vi "Main5states_decoupled.vi"() -> ()   [LabVIEW 2021]
uses:
  controls/SynchroCheckCentral.ctl
  controls/SynchroCheckCentral_Info.ctl
  controls/SynchroCheckCentral_Data.ctl
  controls/3ph Phasor.ctl
  controls/Phasor.ctl
  controls/AFE_froming_Central.ctl
  controls/AFE_froming_Central_Info.ctl
  controls/AFE_froming_Central_Data.ctl
  controls/references.ctl
  controls/Connected_OPF.ctl
  controls/Connected_OPF_Info.ctl
  controls/Connected_OPF_Data.ctl
  controls/PVemulator_Central.ctl
  controls/PVemulator_Central_Info.ctl
  controls/PVemulator_Central_Data.ctl
  controls/measurements.ctl
  controls/measurements_SC.ctl
  controls/SC_references.ctl
  controls/MeteoBoxCentral.ctl
  controls/MeteoBoxCentral_Info.ctl
  controls/MeteoBoxCentral_Data.ctl
  controls/SCADA_to_SM.ctl
  controls/SCADAOGCentral_Info.ctl
  controls/SCADA_to_SM_Data.ctl
  controls/State Machine.ctl
  <vilib>/Platform/TimedLoop/XDataNode/timing_clust.ctl
  <vilib>/Platform/TimedLoop/XDataNode/nitl_modes.ctl
  <vilib>/Platform/TimedLoop/XDataNode/wakeup.ctl
  controls/PV_facade_central.ctl
  controls/PV_facade_cental_Info.ctl
  controls/PV_facade_central_Data.ctl
  controls/state_2.ctl
  <vilib>/Analysis/baseanly.llb/Mean (DBL).vi
  <vilib>/JDP Science/JSONtext/Next JSON Value.vi
  <vilib>/JDP Science/JSONtext/String Subset.vi
  <vilib>/JDP Science/JSONtext/Parsing/Advance past next JSON Value (inlined COPY).vi
  <vilib>/JDP Science/JSONtext/Parsing/Advance past whitespace.vi
  <vilib>/JDP Science/JSONtext/Parsing/Advance past String.vi
  <vilib>/JDP Science/JSONtext/Parsing/Advance past Number.vi
  <vilib>/JDP Science/JSONtext/Parsing/Advance past Line Ending.vi
  <vilib>/Utility/file.llb/Read Delimited Spreadsheet (DBL).vi
  <vilib>/JDP Science/JSONtext/Parsing/Parse Full Path or Item Name.vi
  <vilib>/JDP Science/JSONtext/Parsing/Advance past Array.vi
  <vilib>/JDP Science/JSONtext/Parsing/Advance past Object.vi
  <vilib>/JDP Science/JSONtext/support/Error Cluster From Code.vi
  <vilib>/JDP Science/JSONtext/Offset/Find Item Locations by Path.vi
  <vilib>/Platform/TimedLoop/XDataNode/XDataNode.xnode
  <vilib>/JDP Science/JSONtext/JSONtext.lvlib
  <userlib>/_OpenG.lib/boolean/boolean.llb/openg_boolean__ogtk.lvlib
  <vilib>/Platform/TimedLoop/XDataNode/XDNodeRunTimeDep.lvlib
  <vilib>/Analysis/NI_AALBase.lvlib
panel:
  out "old_sp_island_bool":bool=TRUE
  out "old_sp_island":dbl[](array[numeric])
  out "V_freq_for_island":dbl
  out "V_freq":dbl
  out "V angle":cluster{"output":dbl}(graph)
  in  "Reset_angle":bool
  out "SOC":cluster{"mean":dbl}(graph)
  out "V_control_fix_for_island":dbl
  out "V control":cluster{"output":dbl}(graph)
  out "V_control":dbl
  out "V_afe":dbl
  out "V_upstream":dbl
  in  "Reset_magnitude":bool
  out "SCADA data":bool
  in  "SCADA":T1={"Info"={"Resource"="MeteoBox", "Problem"=FALSE, "Timestamp"=0.0}, "Data"={"Voltage mag"=[], "Voltage angle"=[]}}
  in  "to connected-island":bool
  in  "Real_SOC":bool
  out "P_pv_facade":dbl
  in  "SOC":dbl=50.0
  in  "IN Meteo":T4={"Info"={"Resource"="MeteoBox", "Problem"=FALSE, "Timestamp"=0.0}, "Data"={"GI"=0.0, "GHI"=0.0, "GVI"=0.0, "Tair"=0.0, "Tcell roof"=0.0, "Global_Total_Irr"=0.0, "Diffused_Irr"=0.0, "Tcell facade"=0.0, "PV_mpp"={"perun"=0.0, "solarmax"=0.0, "facade"=0.0, "emul4"=0.0, "emul5"=0.0, "emul6"=0.0, "emul7"=0.0}}}
  out "SC_soc":dbl
  out "delta angle":dbl
  in  "Send sp DC?":bool
  in  "Send sp AC?":bool
  out "Zenone_Q":dbl
  out "Zenone_P":dbl
  out "forming SC?":bool
  out "OUT PV+SC":T7={"Info"={"Resource"="Zenone", "Problem"=FALSE, "Timestamp"=0.0}, "Data"={"Status 1"=FALSE, "Status 2"=FALSE, "measurements"={"V_PV1"=0.0, "V_CAP1"=0.0, "V_PV2"=0.0, "V_CAP2"=0.0, "V_grid2"=0.0, "V_PV3"=0.0, "V_CAP3"=0.0, "V_grid3"=0.0, "V_PV4"=0.0, "V_CAP4"=0.0, "V_grid4"=0.0, "V_grid1"=0.0, "P1"=0.0, "P2"=0.0, "P3"=0.0, "P4"=0.0}, "Status 3"=FALSE, "Status 4"=FALSE, "measurements SC"={"V_SC"=0.0, "V_CAP"=0.0, "V_grid"=0.0, "P"=0.0, "SOC"=0.0}, "Status SC"=FALSE, "Forming/Following"=FALSE, "Start forming"=FALSE, "SC references"={"Vdc"=0.0, "Pdc"=0.0}, "Start following"=FALSE}}
  out "PV data":bool
  out "AFE data":bool
  out "synchro data":bool
  in  "IN PV+SC":T7={"Info"={"Resource"="Zenone", "Problem"=FALSE, "Timestamp"=0.0}, "Data"={"Status 1"=FALSE, "Status 2"=FALSE, "measurements"={"V_PV1"=0.0, "V_CAP1"=0.0, "V_PV2"=0.0, "V_CAP2"=0.0, "V_grid2"=0.0, "V_PV3"=0.0, "V_CAP3"=0.0, "V_grid3"=0.0, "V_PV4"=0.0, "V_CAP4"=0.0, "V_grid4"=0.0, "V_grid1"=0.0, "P1"=0.0, "P2"=0.0, "P3"=0.0, "P4"=0.0}, "Status 3"=FALSE, "Status 4"=FALSE, "measurements SC"={"V_SC"=0.0, "V_CAP"=0.0, "V_grid"=0.0, "P"=0.0, "SOC"=0.0}, "Status SC"=FALSE, "Forming/Following"=FALSE, "Start forming"=FALSE, "SC references"={"Vdc"=0.0, "Pdc"=0.0}, "Start following"=FALSE}}
  out "iOPF data":bool
  out "cOPF data":bool
  in  "IN AFE":T13={"Info"={"Resource"="Zenone", "Problem"=FALSE, "Timestamp"=0.0}, "Data"={"Start forming 1"=FALSE, "Forming/Following"=[], "Start forming 2"=FALSE, "measurements"={"Vdc1"=0.0, "P1"=0.0, "Vdc2"=0.0, "P2"=0.0, "Q2"=0.0, "Vdc3"=0.0, "P3"=0.0, "Q3"=0.0, "Vdc4"=0.0, "P4"=0.0, "Q4"=0.0, "Q1"=0.0}, "Status"=[], "references"={"Vdc1"=0.0, "Vdc2"=0.0, "Qac2"=0.0, "Vdc3"=0.0, "Qac3"=0.0, "Vdc4"=0.0, "Qac4"=0.0, "Qac1"=0.0, "V_arg2"=0.0, "V_abs2"=0.0, "V_abs1"=0.0, "V_arg1"=0.0, "freq1"=0.0, "freq2"=0.0}, "Start following 1"=FALSE, "Start following 2"=FALSE}}
  in  "IN cOPF":T17={"Info"={"Resource"="Zenone", "Problem"=0.0, "Timestamp"=0.0}, "Data"={"Operation_mode"="Grid connected", "solution_feasible"=0.0, "Optimal_slack"="AFE 1", "setpoints"=[], "upper_layer_grid_info"={"Frequency"=0.0, "Angle"=0.0, "Magnitude"=0.0}, "SC_soc"=0.0, "PV"={"perun"=0.0, "solarmax"=0.0, "facade"=0.0, "emul4"=0.0, "emul5"=0.0, "emul6"=0.0, "emul7"=0.0}, "P_pv_facade"=0.0}}
  in  "IN iOPF":T17={"Info"={"Resource"="Zenone", "Problem"=0.0, "Timestamp"=0.0}, "Data"={"Operation_mode"="Grid connected", "solution_feasible"=0.0, "Optimal_slack"="AFE 1", "setpoints"=[], "upper_layer_grid_info"={"Frequency"=0.0, "Angle"=0.0, "Magnitude"=0.0}, "SC_soc"=0.0, "PV"={"perun"=0.0, "solarmax"=0.0, "facade"=0.0, "emul4"=0.0, "emul5"=0.0, "emul6"=0.0, "emul7"=0.0}, "P_pv_facade"=0.0}}
  in  "IN synchro":T20={"Info"={"Resource"="SyncroCheck", "Problem"=FALSE, "Timestamp"=0.0}, "Data"={"close/open relay"=TRUE, "Operation mode"="Grid connected", "V_Downstream"={"Phase A"={"Frequency"=0.0, "Magnitude"=0.0, "Angle [Deg]"=0.0}, "Phase B"={"Frequency"=0.0, "Magnitude"=0.0, "Angle [Deg]"=0.0}, "Phase C"={"Frequency"=0.0, "Magnitude"=0.0, "Angle [Deg]"=0.0}, "Phase N"={"Frequency"=0.0, "Magnitude"=0.0, "Angle [Deg]"=0.0}}, "V_UpStream"={"Phase A"={"Frequency"=0.0, "Magnitude"=0.0, "Angle [Deg]"=0.0}, "Phase B"={"Frequency"=0.0, "Magnitude"=0.0, "Angle [Deg]"=0.0}, "Phase C"={"Frequency"=0.0, "Magnitude"=0.0, "Angle [Deg]"=0.0}, "Phase N"={"Frequency"=0.0, "Magnitude"=0.0, "Angle [Deg]"=0.0}}, "Synchronised?"=TRUE}}
  out "OUT iOPF":T17={"Info"={"Resource"="Zenone", "Problem"=0.0, "Timestamp"=0.0}, "Data"={"Operation_mode"="Grid connected", "solution_feasible"=0.0, "Optimal_slack"="AFE 1", "setpoints"=[], "upper_layer_grid_info"={"Frequency"=0.0, "Angle"=0.0, "Magnitude"=0.0}, "SC_soc"=0.0, "PV"={"perun"=0.0, "solarmax"=0.0, "facade"=0.0, "emul4"=0.0, "emul5"=0.0, "emul6"=0.0, "emul7"=0.0}, "P_pv_facade"=0.0}}
  out "OUT cOPF":T17={"Info"={"Resource"="Zenone", "Problem"=0.0, "Timestamp"=0.0}, "Data"={"Operation_mode"="Grid connected", "solution_feasible"=0.0, "Optimal_slack"="AFE 1", "setpoints"=[], "upper_layer_grid_info"={"Frequency"=0.0, "Angle"=0.0, "Magnitude"=0.0}, "SC_soc"=0.0, "PV"={"perun"=0.0, "solarmax"=0.0, "facade"=0.0, "emul4"=0.0, "emul5"=0.0, "emul6"=0.0, "emul7"=0.0}, "P_pv_facade"=0.0}}
  out "OUT AFE":T13={"Info"={"Resource"="Zenone", "Problem"=FALSE, "Timestamp"=0.0}, "Data"={"Start forming 1"=FALSE, "Forming/Following"=[], "Start forming 2"=FALSE, "measurements"={"Vdc1"=0.0, "P1"=0.0, "Vdc2"=0.0, "P2"=0.0, "Q2"=0.0, "Vdc3"=0.0, "P3"=0.0, "Q3"=0.0, "Vdc4"=0.0, "P4"=0.0, "Q4"=0.0, "Q1"=0.0}, "Status"=[], "references"={"Vdc1"=0.0, "Vdc2"=0.0, "Qac2"=0.0, "Vdc3"=0.0, "Qac3"=0.0, "Vdc4"=0.0, "Qac4"=0.0, "Qac1"=0.0, "V_arg2"=0.0, "V_abs2"=0.0, "V_abs1"=0.0, "V_arg1"=0.0, "freq1"=0.0, "freq2"=0.0}, "Start following 1"=FALSE, "Start following 2"=FALSE}}
  out "OUT Synchro":T20={"Info"={"Resource"="SyncroCheck", "Problem"=FALSE, "Timestamp"=0.0}, "Data"={"close/open relay"=TRUE, "Operation mode"="Grid connected", "V_Downstream"={"Phase A"={"Frequency"=0.0, "Magnitude"=0.0, "Angle [Deg]"=0.0}, "Phase B"={"Frequency"=0.0, "Magnitude"=0.0, "Angle [Deg]"=0.0}, "Phase C"={"Frequency"=0.0, "Magnitude"=0.0, "Angle [Deg]"=0.0}, "Phase N"={"Frequency"=0.0, "Magnitude"=0.0, "Angle [Deg]"=0.0}}, "V_UpStream"={"Phase A"={"Frequency"=0.0, "Magnitude"=0.0, "Angle [Deg]"=0.0}, "Phase B"={"Frequency"=0.0, "Magnitude"=0.0, "Angle [Deg]"=0.0}, "Phase C"={"Frequency"=0.0, "Magnitude"=0.0, "Angle [Deg]"=0.0}, "Phase N"={"Frequency"=0.0, "Magnitude"=0.0, "Angle [Deg]"=0.0}}, "Synchronised?"=TRUE}}
  out "setpoints":dbl[](array[numeric])
  in  "nb instances":i16=7
  out "optimal_slack":string(combo)="AFE 1"
  out "iOPF valid":bool
  out "forming AFE?":bool
  out "cOPF valid?":bool
  out "synchronised?":bool
  in  "to grid connection":bool
  in  "to prepare for grid connection":bool
  in  "to island":bool
  in  "Stop":bool
  in  "to prepare for island":bool
  # "32.58"
  # "Islanding Manoeuvre - State Machine"
  # "synchronised"
  # "opf connected OK"
  # "opf island OK"
  # "forming AFE?"
  # "forming SC?"
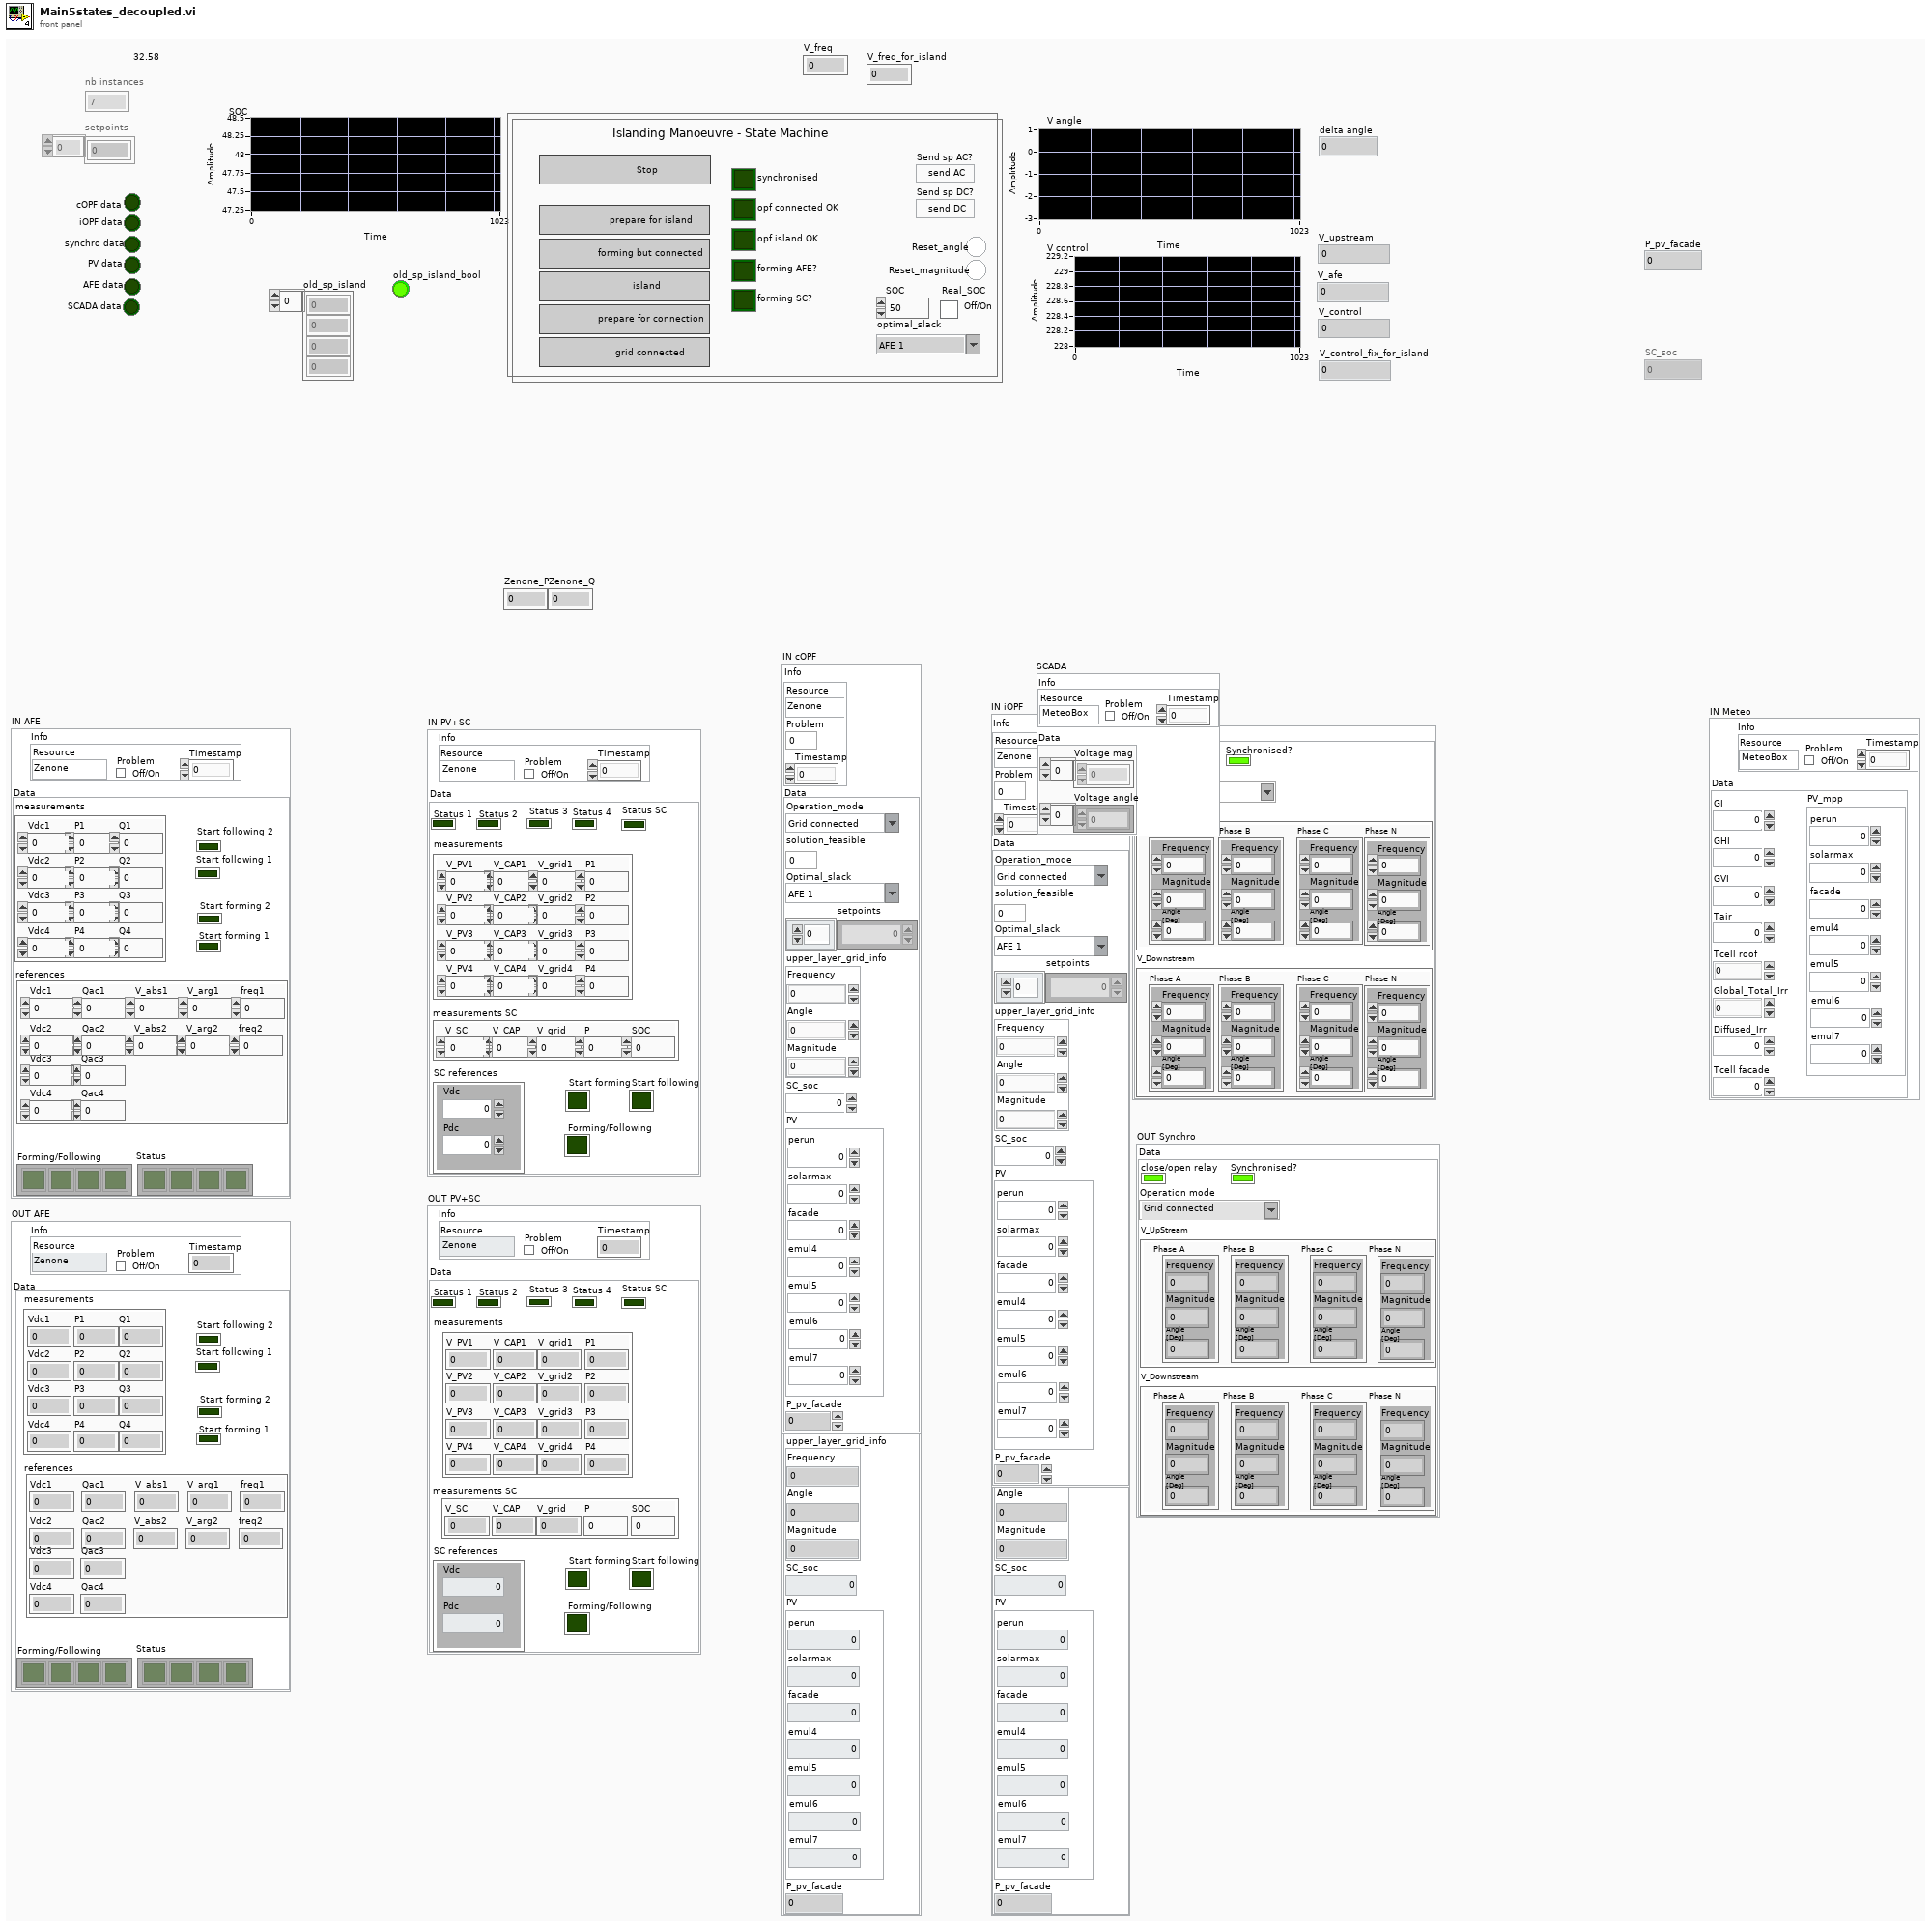
[diagram p1: front panel]
types:
  T1 = typedef "SCADA_to_SM.ctl" = cluster{"Info":T2, "Data":T3}
  T2 = typedef "SCADAOGCentral_Info.ctl" = cluster{"Resource":string, "Problem":bool, "Timestamp":dbl}
  T3 = typedef "SCADA_to_SM_Data.ctl" = cluster{"Voltage mag":dbl[], "Voltage angle":dbl[]}
  T4 = typedef "MeteoBoxCentral.ctl" = cluster{"Info":T5, "Data":T6}
  T5 = typedef "MeteoBoxCentral_Info.ctl" = cluster{"Resource":string, "Problem":bool, "Timestamp":dbl}
  T6 = typedef "MeteoBoxCentral_Data.ctl" = cluster{"GI":dbl, "GHI":dbl, "GVI":dbl, "Tair":dbl, "Tcell roof":dbl, "Global_Total_Irr":dbl, "Diffused_Irr":dbl, "Tcell facade":dbl, "PV_mpp":cluster{"perun":dbl, "solarmax":dbl, "facade":dbl, "emul4":dbl, "emul5":dbl, "emul6":dbl, "emul7":dbl}}
  T7 = typedef "PVemulator_Central.ctl" = cluster{"Info":T8, "Data":T9}
  T8 = typedef "PVemulator_Central_Info.ctl" = cluster{"Resource":string, "Problem":bool, "Timestamp":dbl}
  T9 = typedef "PVemulator_Central_Data.ctl" = cluster{"Status 1":bool, "Status 2":bool, "measurements":T10, "Status 3":bool, "Status 4":bool, "measurements SC":T11, "Status SC":bool, "Forming/Following":bool, "Start forming":bool, "SC references":T12, "Start following":bool}
  T10 = typedef "measurements.ctl" = cluster{"V_PV1":dbl, "V_CAP1":dbl, "V_PV2":dbl, "V_CAP2":dbl, "V_grid2":dbl, "V_PV3":dbl, "V_CAP3":dbl, "V_grid3":dbl, "V_PV4":dbl, "V_CAP4":dbl, "V_grid4":dbl, "V_grid1":dbl, "P1":dbl, "P2":dbl, "P3":dbl, "P4":dbl}
  T11 = typedef "measurements_SC.ctl" = cluster{"V_SC":dbl, "V_CAP":dbl, "V_grid":dbl, "P":dbl, "SOC":dbl}
  T12 = typedef "SC_references.ctl" = cluster{"Vdc":dbl, "Pdc":dbl}
  T13 = typedef "AFE_froming_Central.ctl" = cluster{"Info":T14, "Data":T15}
  T14 = typedef "AFE_froming_Central_Info.ctl" = cluster{"Resource":string, "Problem":bool, "Timestamp":dbl}
  T15 = typedef "AFE_froming_Central_Data.ctl" = cluster{"Start forming 1":bool, "Forming/Following":bool[], "Start forming 2":bool, "measurements":cluster{"Vdc1":dbl, "P1":dbl, "Vdc2":dbl, "P2":dbl, "Q2":dbl, "Vdc3":dbl, "P3":dbl, "Q3":dbl, "Vdc4":dbl, "P4":dbl, "Q4":dbl, "Q1":dbl}, "Status":bool[], "references":T16, "Start following 1":bool, "Start following 2":bool}
  T16 = typedef "references.ctl" = cluster{"Vdc1":dbl, "Vdc2":dbl, "Qac2":dbl, "Vdc3":dbl, "Qac3":dbl, "Vdc4":dbl, "Qac4":dbl, "Qac1":dbl, "V_arg2":dbl, "V_abs2":dbl, "V_abs1":dbl, "V_arg1":dbl, "freq1":dbl, "freq2":dbl}
  T17 = typedef "Connected_OPF.ctl" = cluster{"Info":T18, "Data":T19}
  T18 = typedef "Connected_OPF_Info.ctl" = cluster{"Resource":string, "Problem":dbl, "Timestamp":dbl}
  T19 = typedef "Connected_OPF_Data.ctl" = cluster{"Operation_mode":string, "solution_feasible":dbl, "Optimal_slack":string, "setpoints":dbl[], "upper_layer_grid_info":cluster{"Frequency":dbl, "Angle":dbl, "Magnitude":dbl}, "SC_soc":dbl, "PV":cluster{"perun":dbl, "solarmax":dbl, "facade":dbl, "emul4":dbl, "emul5":dbl, "emul6":dbl, "emul7":dbl}, "P_pv_facade":dbl}
  T20 = typedef "SynchroCheckCentral.ctl" = cluster{"Info":T21, "Data":T22}
  T21 = typedef "SynchroCheckCentral_Info.ctl" = cluster{"Resource":string, "Problem":bool, "Timestamp":dbl}
  T22 = typedef "SynchroCheckCentral_Data.ctl" = cluster{"close/open relay":bool, "Operation mode":string, "V_Downstream":T23, "V_UpStream":T23, "Synchronised?":bool}
  T23 = typedef "3ph Phasor.ctl" = cluster{"Phase A":T24, "Phase B":T24, "Phase C":T24, "Phase N":T24}
  T24 = typedef "Phasor.ctl" = cluster{"Frequency":dbl, "Magnitude":dbl, "Angle [Deg]":dbl}
  T25 = typedef "State Machine.ctl" = enum16{"Grid connected", "Prepare for island", "Forming but connected", "Island", "Prepare for connection"}
  T26 = typedef "XDNodeRunTimeDep.lvlib/timing_clust.ctl" = cluster{"Expected End [f-1]":u64, "Actual End [f-1]":u64, "Finished Late? [f-1]":bool, "Expected End [i-1]":u64, "Actual End [i-1]":u64, "Finished Late? [i-1]":bool, "Expected Start [i]":u64, "Actual Start [i]":u64, "Expected Start [f]":u64, "Actual Start [f]":u64, "Source Name":string, "Structure Name":string, "Period":i64, "Deadline":i64, "Offset":i64, "Start":i64, "Priority":i32, "Timeout":i32, "Mode":T27, "Wakeup Reason":T28, "Error":errorcluster, "Source Type":string, "Secondary Source Type":string, "Global End Time":u64, "Global Start Time":u64, "Frame Duration":u64, "Iteration Duration":u64, "Assigned CPU":i32, "I/O Scan Engine Mode":u32}
  T27 = typedef "XDNodeRunTimeDep.lvlib/nitl_modes.ctl" = enum32{"No Change", "Process missed periods, maintain original phase", "Discard missed periods, maintain original phase", "Process missed periods, ignore original phase", "Discard missed periods, ignore original phase"}
  T28 = typedef "XDNodeRunTimeDep.lvlib/wakeup.ctl" = enum32{"Normal", "Aborted", "Asynchronous wakeup", "Timing source error", "Timed loop error", "Timeout"}
  T29 = typedef "state_2.ctl" = string
  T30 = cluster{"Frequency":dbl, "Angle":dbl, "Magnitude":dbl}
  T31 = cluster{"perun":dbl, "solarmax":dbl, "facade":dbl, "emul4":dbl, "emul5":dbl, "emul6":dbl, "emul7":dbl}
  T32 = typedef "PV_facade_central.ctl" = cluster{"Info":T33, "Data":T34}
  T33 = typedef "PV_facade_cental_Info.ctl" = cluster{"Resource":string, "Problem":bool, "Timestamp":dbl}
  T34 = typedef "PV_facade_central_Data.ctl" = cluster{"P":dbl, "Q":dbl, "Pset":dbl, "Qset":dbl}
  T35 = typedef "Setpoints_CDA.ctl" = cluster{"ZENONE":T36, "BESS":T36, "PERUN":T36, "SOLMAX":T36}
  T36 = typedef "Setpoints_CDA_ZENONE.ctl" = cluster{"P_set [kW]":dbl, "Q_set [kVAr]":dbl}
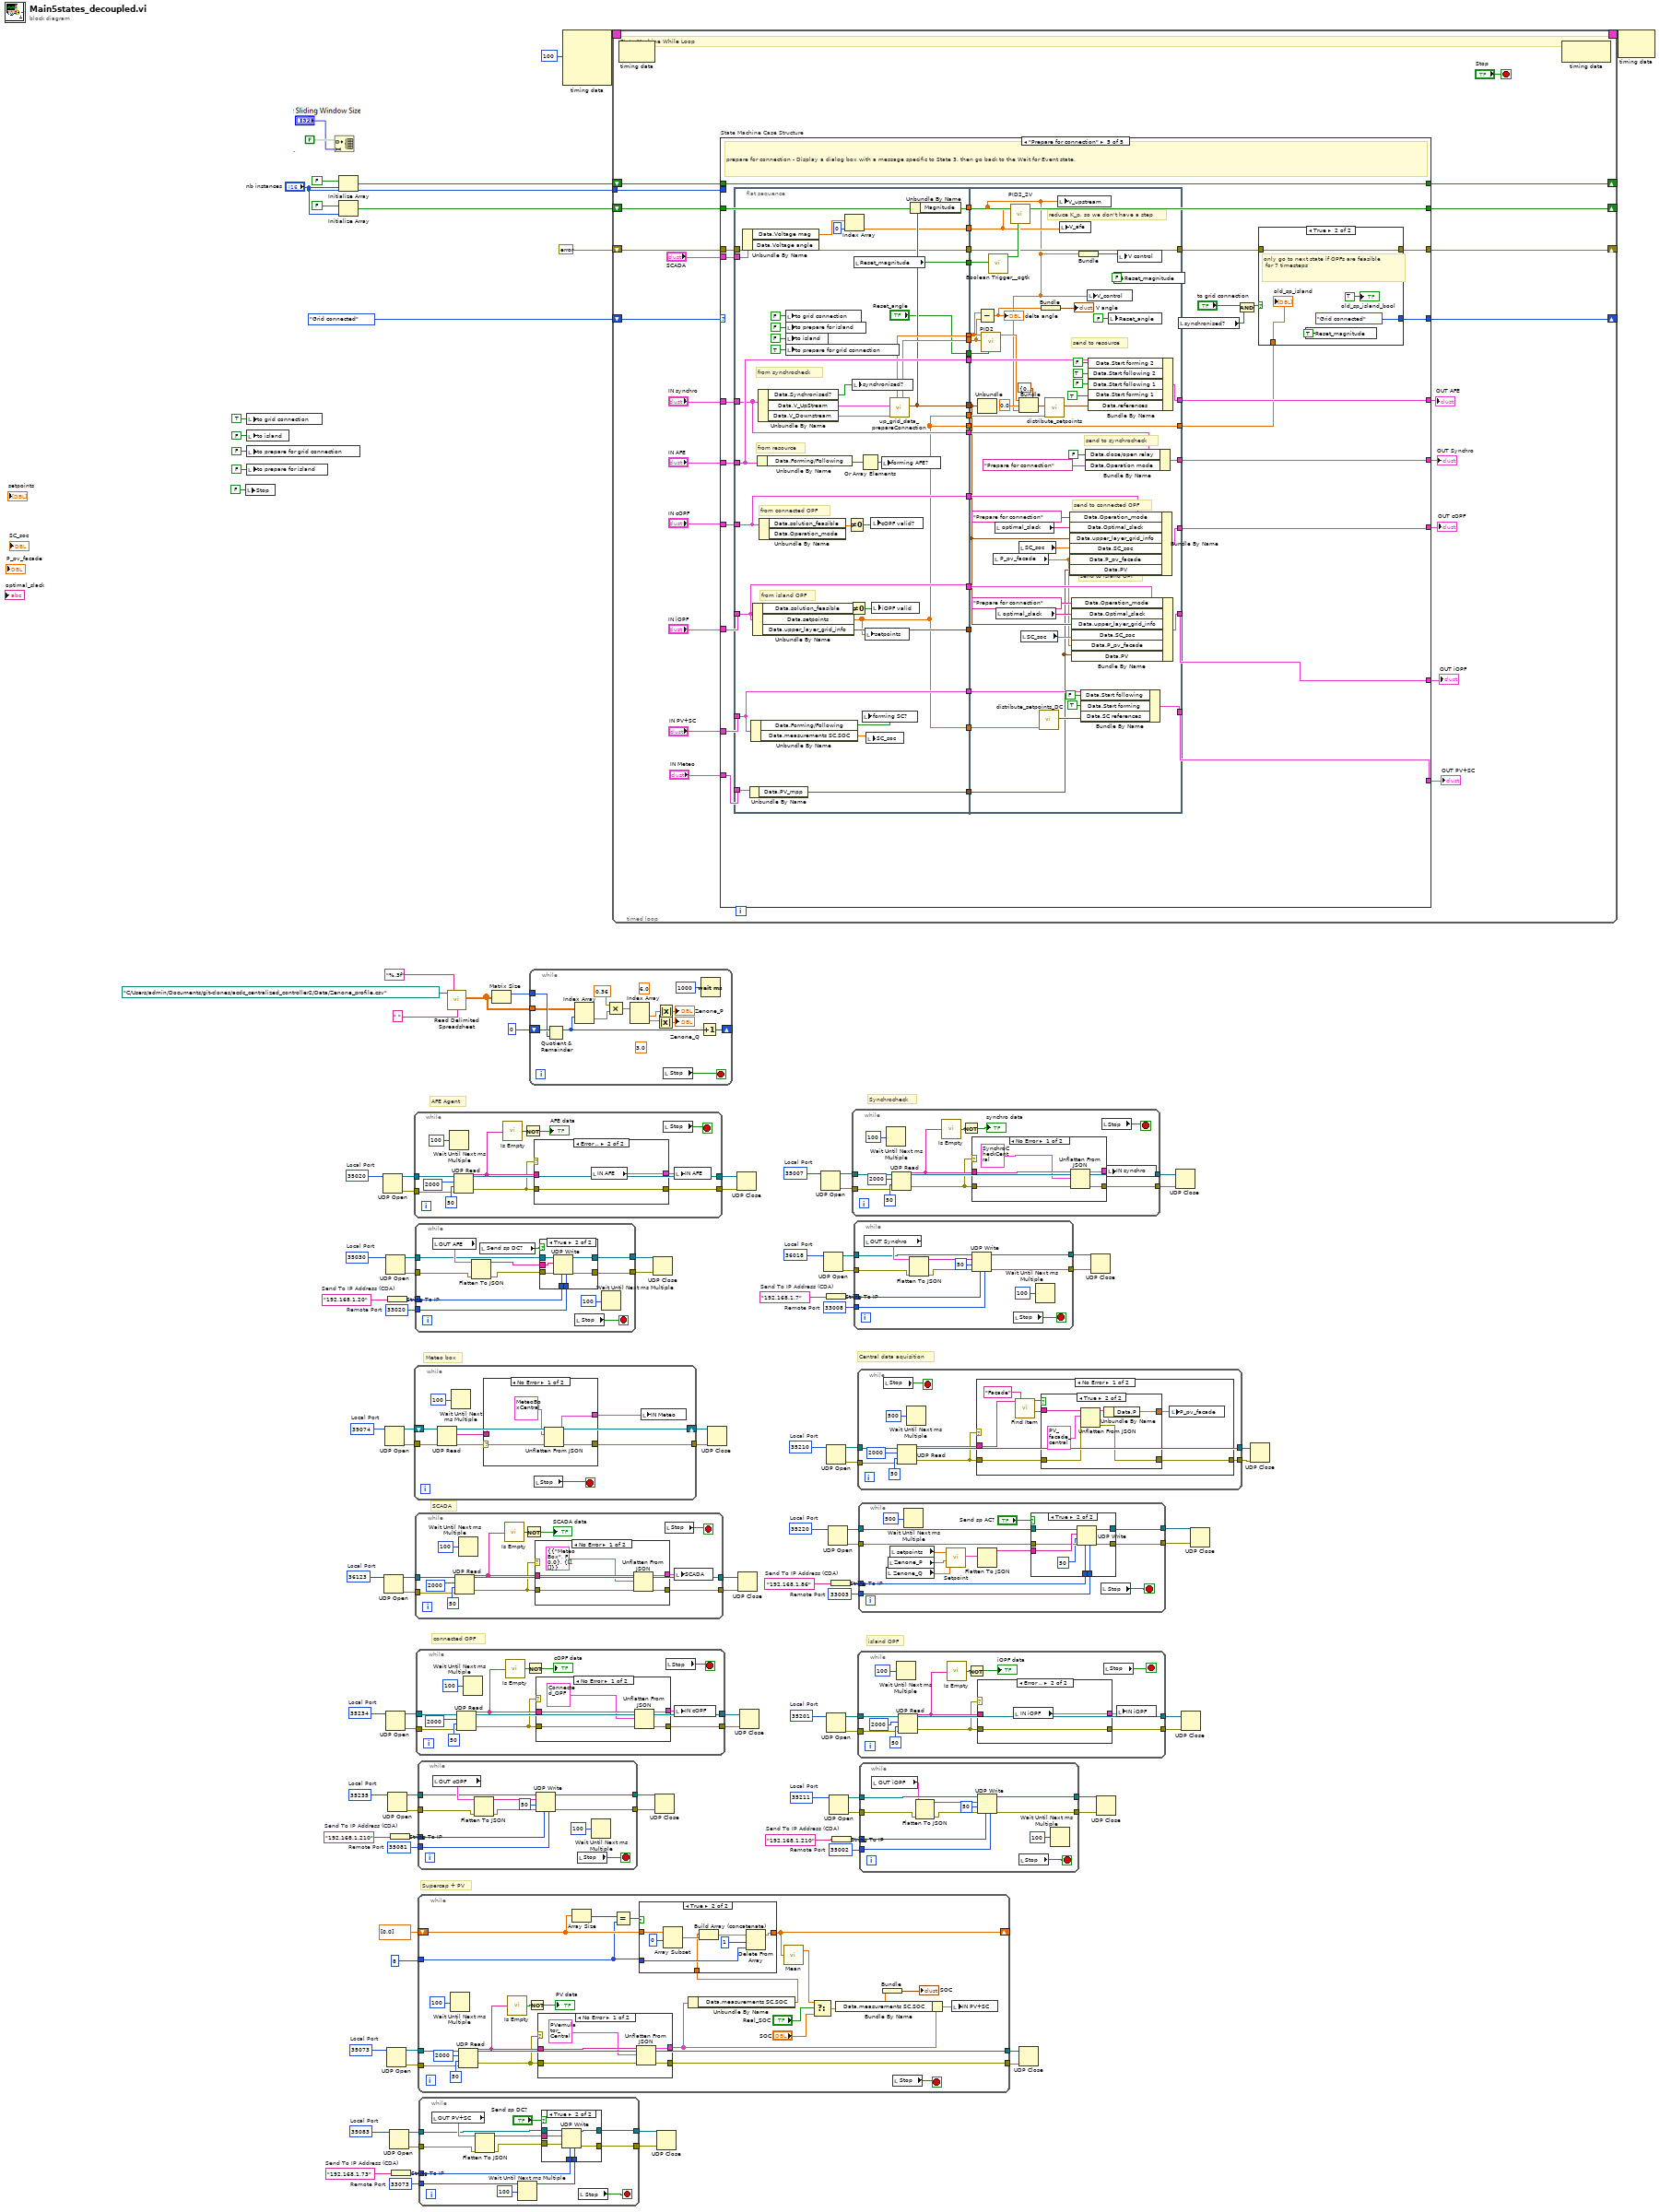
[diagram p0: block diagram]
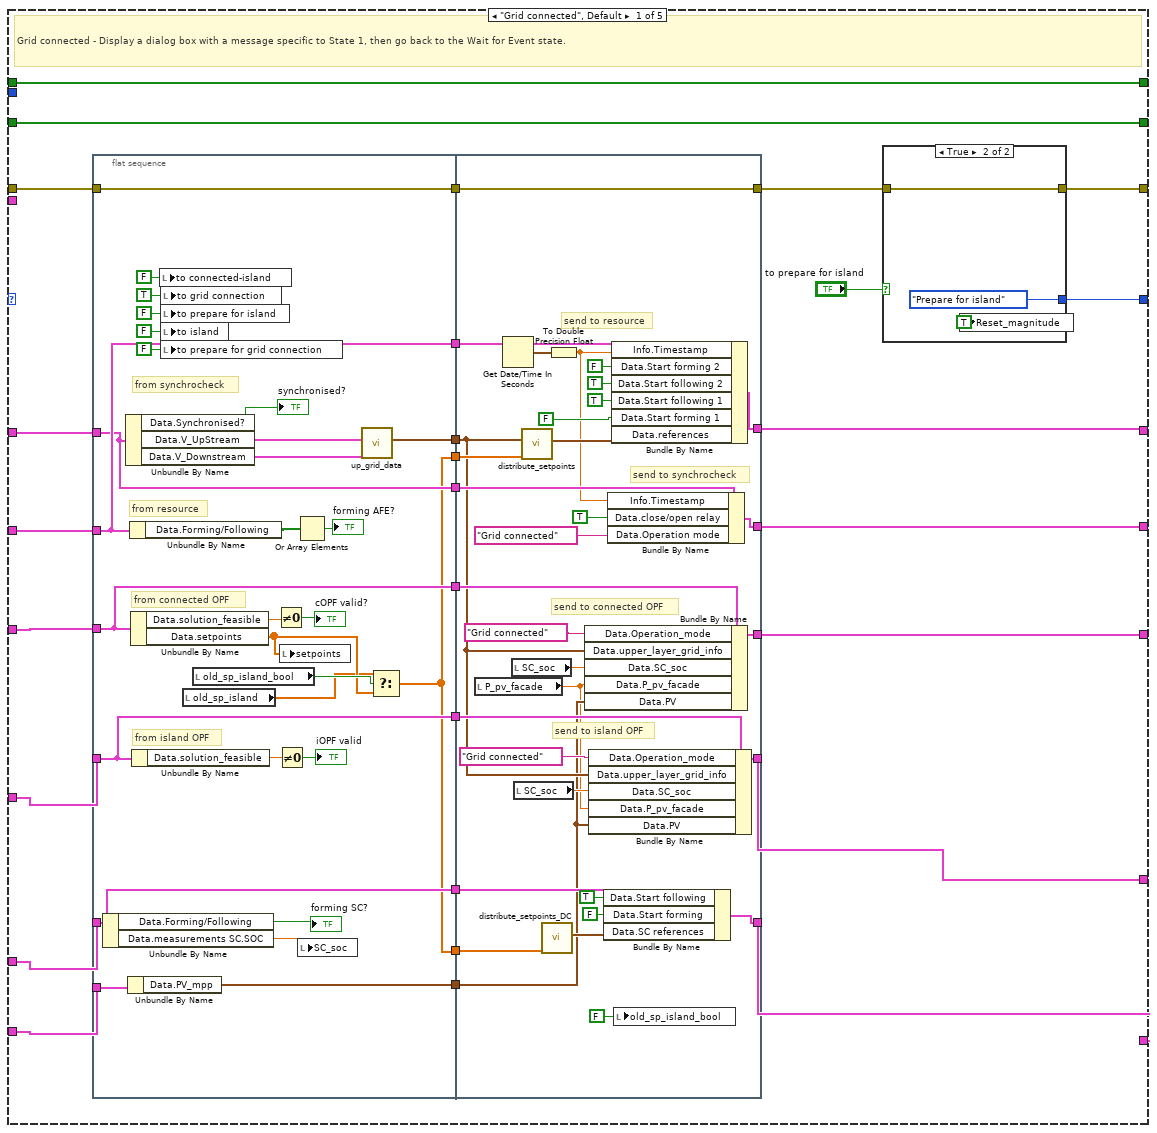
[diagram p2: hidden frame]
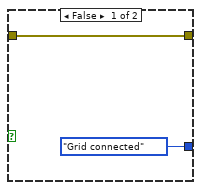
[diagram p3: hidden frame]
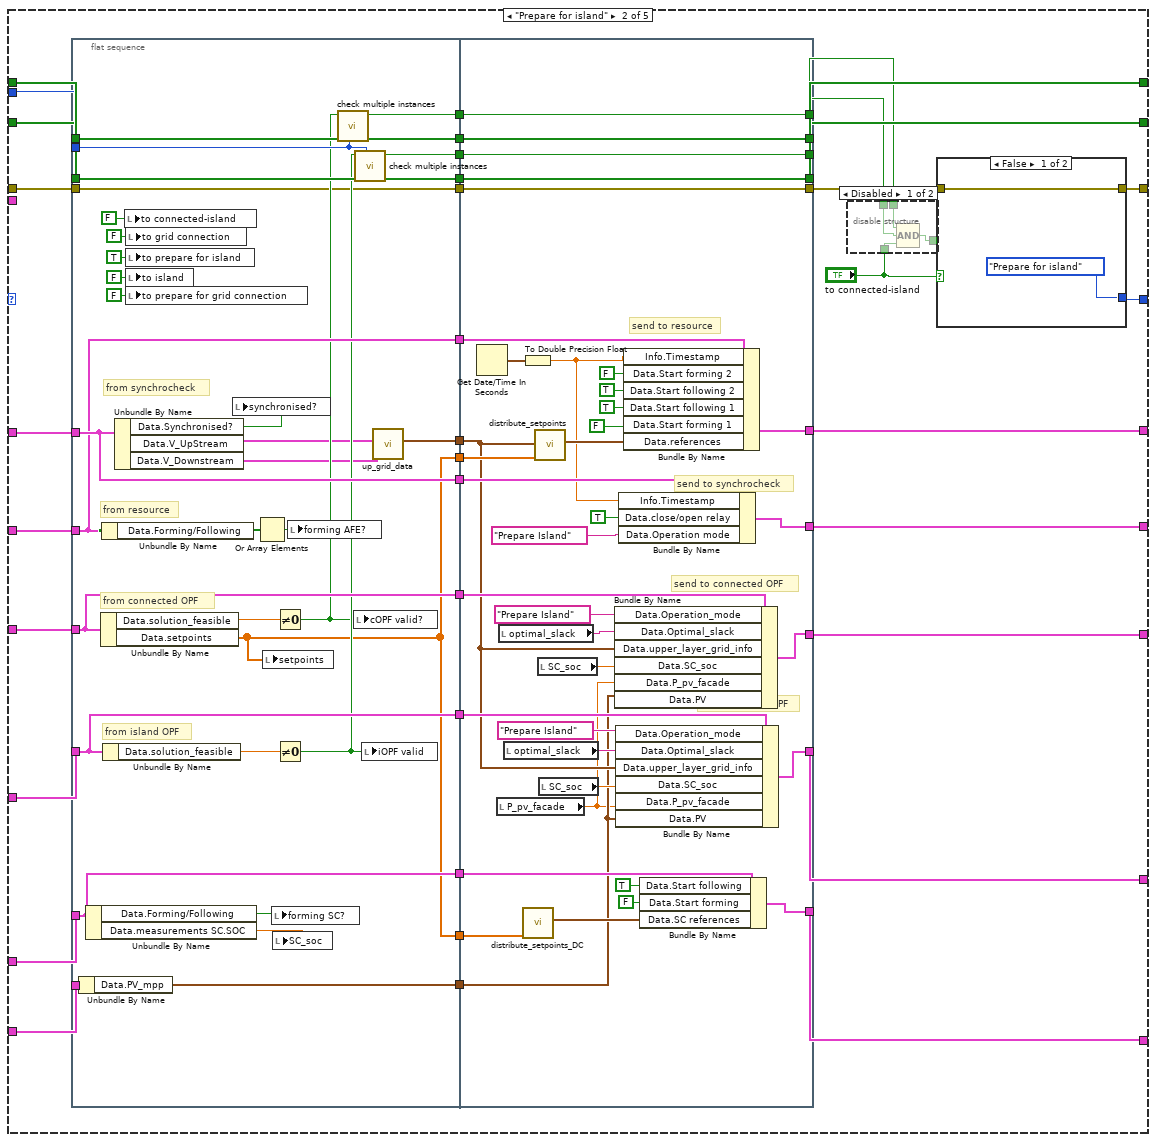
[diagram p4: hidden frame]
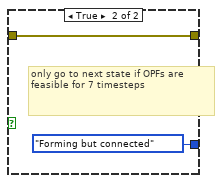
[diagram p6: hidden frame]
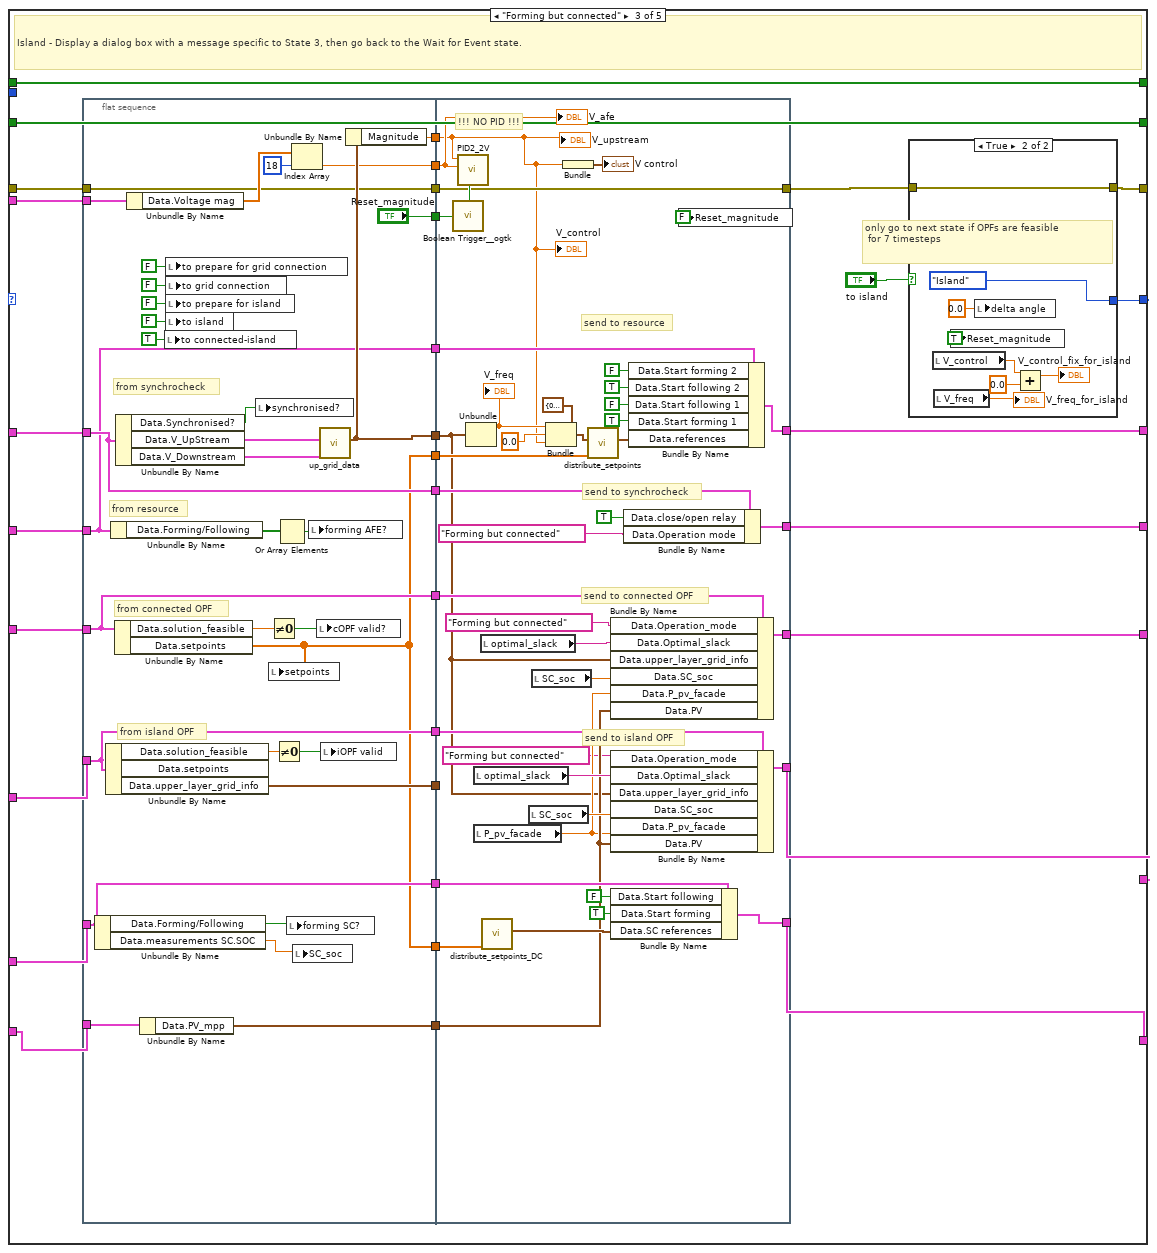
[diagram p7: hidden frame]
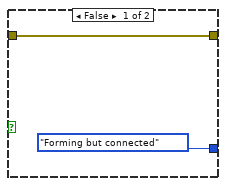
[diagram p8: hidden frame]
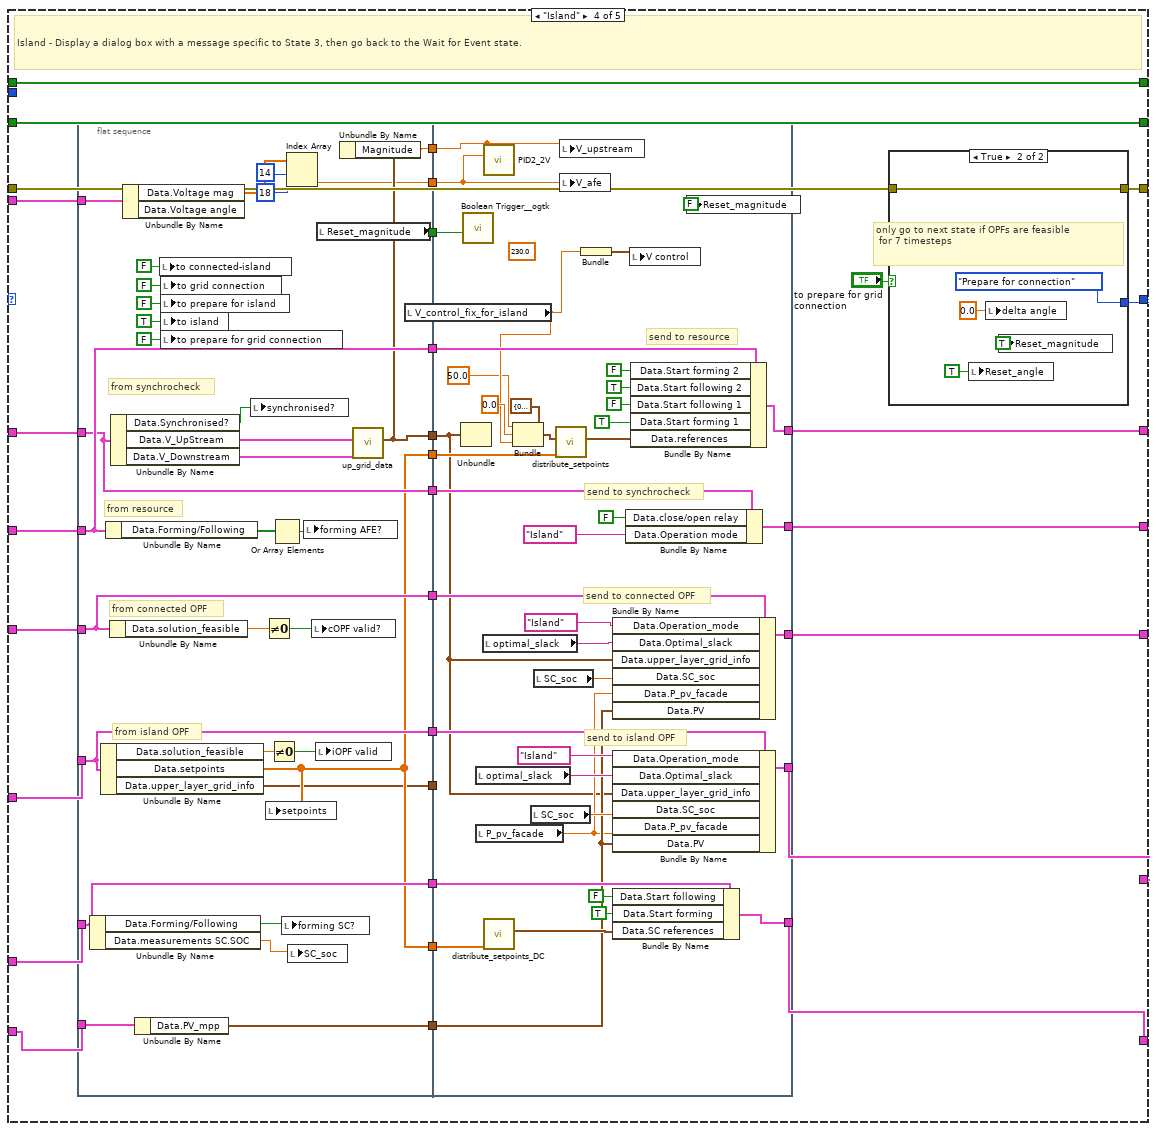
[diagram p9: hidden frame]
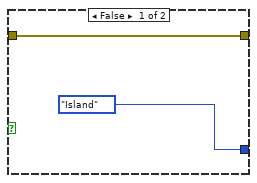
[diagram p10: hidden frame]
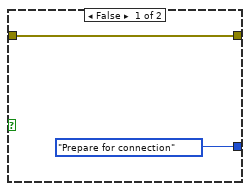
[diagram p11: hidden frame]
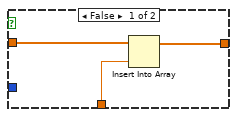
[diagram p12: hidden frame]
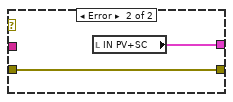
[diagram p13: hidden frame]
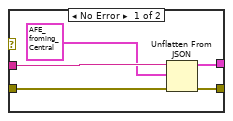
[diagram p16: hidden frame]
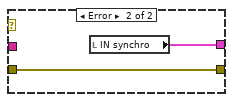
[diagram p17: hidden frame]
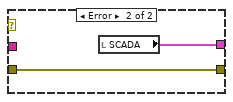
[diagram p18: hidden frame]
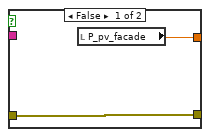
[diagram p20: hidden frame]
diagram:
  w10 = u16 35083  # Local Port
  w12 = u16 33073  # Remote Port
  w13 = "192.168.1.73"  # Send To IP Address (CDA)
  w14 = u16 35073  # Local Port
  w23 = u16 35030  # Local Port
  w25 = u16 33020  # Remote Port
  w26 = "192.168.1.20"  # Send To IP Address (CDA)
  w27 = u16 35020  # Local Port
  w35 = u16 36018  # Local Port
  w32 = u16 33008  # Remote Port
  w34 = "192.168.1.7"  # Send To IP Address (CDA)
  w33 = u16 35007  # Local Port
  w45 = u16 36123  # Local Port
  w54 = u16 35220  # Local Port
  w56 = u16 33003  # Remote Port
  w57 = "192.168.1.86"  # Send To IP Address (CDA)
  w58 = u16 35210  # Local Port
  w65 = u16 35211  # Local Port
  w63 = u16 35002  # Remote Port
  w64 = "192.168.1.210"  # Send To IP Address (CDA)
  w66 = u16 35201  # Local Port
  w80 = u16 35235  # Local Port
  w82 = u16 35081  # Remote Port
  w83 = "192.168.1.210"  # Send To IP Address (CDA)
  w84 = u16 35234  # Local Port
  w95 = u16 39074  # Local Port
  # "Supercap + PV"
  # "AFE Agent"
  # "Synchrocheck"
  # "SCADA"
  # "Meteo box"
  # "Central data aquisition"
  # "connected OPF"
  # "island OPF"
  n1 = local write "Stop"(FALSE ("Stop")) -> ()
  n2 = local write "to grid connection"(TRUE ("to grid connection")) -> ()
  n3 = local write "to island"(FALSE ("to island")) -> ()
  n4 = local write "to prepare for grid connection"(FALSE ("to prepare for grid connection")) -> ()
  n5 = local write "to prepare for island"(FALSE ("to prepare for island")) -> ()
  n6 = Initialize Array(FALSE, "nb instances") -> (w110:bool[])
  n7 = Initialize Array(FALSE, "nb instances") -> (w108:bool[])
  n8 = UDP Open(11:w27) -> (port=w29:refnum<k16>, 0:w28:errorcluster)  [unwired: 4 in, 1 out]
  n9 = UDP Open(11:w45) -> (port=w47:refnum<k16>, 0:w46:errorcluster)  [unwired: 4 in, 1 out]
  n10 = UDP Open(11:w95) -> (port=w94:refnum<k16>, 0:w93:errorcluster)  [unwired: 4 in, 1 out]
  n11 = UDP Open(11:w23) -> (port=w20:refnum<k16>, 0:w19:errorcluster)  [unwired: 4 in, 1 out]
  n12 = UDP Open(11:w84) -> (port=w86:refnum<k16>, 0:w85:errorcluster)  [unwired: 4 in, 1 out]
  n13 = UDP Open(11:w14) -> (port=w16:refnum<k16>, 0:w15:errorcluster)  [unwired: 4 in, 1 out]
  n14 = String To IP(1:w26) -> (0:w24:u32)
  n15 = UDP Open(11:w80) -> (port=w77:refnum<k16>, 0:w76:errorcluster)  [unwired: 4 in, 1 out]
  n16 = UDP Open(11:w10) -> (port=w7:refnum<k16>, 0:w6:errorcluster)  [unwired: 4 in, 1 out]
  n17 = String To IP(1:w83) -> (0:w81:u32)
  n18 = String To IP(1:w13) -> (0:w11:u32)
  n19 = while {
    tunnel: w29 -> [w119]
    tunnel: w28 -> [w118]
    tunnel: [w117] -> w31
    tunnel: [w116] -> w30
    stop <- w122 stop-if-true
    (unwired) i64 0 ("Iteration Duration")
    n20 = Wait Until Next ms Multiple(millisecond multiple=u32 100) -> ()  [unwired: 1 out]
    n21 = UDP Read(connection ID=w119, max size (548)=2000, timeout ms (25000)=50, 8:w118) -> (data out=w120:string, error out=w115:errorcluster, 3:w116:refnum<k16>)  [unwired: 2 out]
    n22 = call <vilib>:"Is Empty.vi"("JSON"=w120) -> ("Empty"=w123:bool)  [unwired: 4 in]
    n23 = Not(x=w123) -> (.not. x?=→"AFE data":bool)
    n24 = case shown="Error .." w115 {
      tunnel: w115 -> [w128 w131]
      tunnel: w120 -> [w127 _]
      tunnel: [w129 w131] -> w117
      tunnel: [w126 w130] -> w121
      frame No Error {
        n25 = Unflatten From JSON(JSON string=w127, type and defaults=T13 {"Info"={"Resource"="Zenone", "Problem"=FALSE, "Timestamp"=0.0}, "Data"={"Start forming 1"=FALSE, "Forming/Following"=[], "Start forming 2"=FALSE, "measurements"={"Vdc1"=0.0, "P1"=0.0, "Vdc2"=0.0, "P2"=0.0, "Q2"=0.0, "Vdc3"=0.0, "P3"=0.0, "Q3"=0.0, "Vdc4"=0.0, "P4"=0.0, "Q4"=0.0, "Q1"=0.0}, "Status"=[], "references"={"Vdc1"=0.0, "Vdc2"=0.0, "Qac2"=0.0, "Vdc3"=0.0, "Qac3"=0.0, "Vdc4"=0.0, "Qac4"=0.0, "Qac1"=0.0, "V_arg2"=0.0, "V_abs2"=0.0, "V_abs1"=0.0, "V_arg1"=0.0, "freq1"=0.0, "freq2"=0.0}, "Start following 1"=FALSE, "Start following 2"=FALSE}} ("IN AFE"), error in (no error)=w128) -> (value=w126:T13, error out=w129:errorcluster)  [unwired: 4 in]
      }
      frame Error {
        n26 = local read "IN AFE"() -> (w130:T13)
      }
    }
    n27 = local read "Stop"() -> (w122:bool)
    n28 = local write "IN AFE"(w121) -> ()
  }
  n29 = while {
    tunnel: w93 -> [w139]
    tunnel: [w136] -> w92
    shift-right: [w135] -> w91
    shift-left: w94 -> [w140]
    stop <- w134 stop-if-true
    n30 = UDP Read(connection ID=w140, 8:w139) -> (data out=w138:string, error out=w133:errorcluster, 3:w135:refnum<k16>)  [unwired: 2 in, 2 out]
    n31 = Wait Until Next ms Multiple(millisecond multiple=u32 100) -> ()  [unwired: 1 out]
    n32 = case shown="No Error" w133 {
      selector: w133 -> [w141 w146]
      tunnel: w138 -> [w145 _]
      tunnel: [w143 w147] -> w137
      tunnel: [w142 w146] -> w136
      frame No Error {
        n33 = Unflatten From JSON(JSON string=w145, type and defaults=T4 {"Info"={"Resource"="MeteoBox", "Problem"=FALSE, "Timestamp"=0.0}, "Data"={"GI"=0.0, "GHI"=0.0, "GVI"=0.0, "Tair"=0.0, "Tcell roof"=0.0, "Global_Total_Irr"=0.0, "Diffused_Irr"=0.0, "Tcell facade"=0.0, "PV_mpp"={"perun"=0.0, "solarmax"=0.0, "facade"=0.0, "emul4"=0.0, "emul5"=0.0, "emul6"=0.0, "emul7"=0.0}}} ("Cluster"), error in (no error)=w141) -> (value=w143:T4, error out=w142:errorcluster)  [unwired: 4 in]
      }
      frame Error {
        n34 = local read "IN Meteo"() -> (w147:T4)
      }
    }
    n35 = local read "Stop"() -> (w134:bool)
    n36 = local write "IN Meteo"(w137) -> ()
  }
  n37 = while {
    tunnel: w25 -> [w151]
    tunnel: w24 -> [w152]
    tunnel: w20 -> [w154]
    tunnel: w19 -> [w158]
    tunnel: [w150] -> w22
    tunnel: [w149] -> w21
    stop <- w157 stop-if-true
    n38 = local read "OUT AFE"() -> (w159:T13)
    n39 = Flatten To JSON(anything=w159, error in (no error)=w158) -> (JSON string=w155:string, 11:w153:errorcluster)  [unwired: 1 in]
    n40 = local read "Send sp DC?"() -> (w156:bool)
    n41 = case shown="True" w156 {
      tunnel: w155 -> [_ w168]
      tunnel: [w160 w167] -> w149
      tunnel: [w161 w166] -> w150
      tunnel: w154 -> [w161 w165]
      tunnel: w153 -> [w160 w162]
      tunnel: w152 -> [_ w164]
      tunnel: w151 -> [_ w163]
      frame False {
      }
      frame True {
        n42 = UDP Write(address=w164, port or service name=w163, connection ID=w165, data in=w168, 8:w162) -> (error out=w167:errorcluster, 3:w166:refnum<k16>)  [unwired: 1 in]
      }
    }
    n43 = local read "Stop"() -> (w157:bool)
    n44 = Wait Until Next ms Multiple(millisecond multiple=u32 100) -> ()  [unwired: 1 out]
  }
  n45 = while {
    tunnel: w47 -> [w177]
    tunnel: w46 -> [w176]
    tunnel: [w175] -> w49
    tunnel: [w174] -> w48
    stop <- w179 stop-if-true
    (unwired) i64 0 ("Iteration Duration")
    n46 = UDP Read(connection ID=w177, max size (548)=2000, timeout ms (25000)=50, 8:w176) -> (data out=w178:string, error out=w173:errorcluster, 3:w174:refnum<k16>)  [unwired: 2 out]
    n47 = Wait Until Next ms Multiple(millisecond multiple=u32 100) -> ()  [unwired: 1 out]
    n48 = call <vilib>:"Is Empty.vi"("JSON"=w178) -> ("Empty"=w180:bool)  [unwired: 4 in]
    n49 = Not(x=w180) -> (.not. x?=→"SCADA data":bool)
    n50 = case shown="No Error" w173 {
      tunnel: w173 -> [w185 w188]
      tunnel: w178 -> [w184 _]
      tunnel: [w186 w188] -> w175
      tunnel: [w183 w187] -> w171
      frame No Error {
        n51 = Unflatten From JSON(JSON string=w184, type and defaults=T1 {"Info"={"Resource"="MeteoBox", "Problem"=FALSE, "Timestamp"=0.0}, "Data"={"Voltage mag"=[], "Voltage angle"=[]}} ("Cluster"), error in (no error)=w185) -> (value=w183:T1, error out=w186:errorcluster)  [unwired: 4 in]
      }
      frame Error {
        n52 = local read "SCADA"() -> (w187:T1)
      }
    }
    n53 = local read "Stop"() -> (w179:bool)
    n54 = local write "SCADA"(w171) -> ()
  }
  n55 = while {
    tunnel: w86 -> [w195]
    tunnel: w85 -> [w194]
    tunnel: [w193] -> w88
    tunnel: [w192] -> w87
    stop <- w198 stop-if-true
    (unwired) i64 0 ("Iteration Duration")
    n56 = UDP Read(connection ID=w195, max size (548)=2000, timeout ms (25000)=50, 8:w194) -> (data out=w196:string, error out=w191:errorcluster, 3:w192:refnum<k16>)  [unwired: 2 out]
    n57 = Wait Until Next ms Multiple(millisecond multiple=u32 100) -> ()  [unwired: 1 out]
    n58 = call <vilib>:"Is Empty.vi"("JSON"=w196) -> ("Empty"=w200:bool)  [unwired: 4 in]
    n59 = Not(x=w200) -> (.not. x?=→"cOPF data":bool)
    n60 = case shown="No Error" w191 {
      tunnel: w191 -> [w205 w208]
      tunnel: w196 -> [w204 _]
      tunnel: [w206 w208] -> w193
      tunnel: [w202 w207] -> w197
      frame No Error {
        n61 = Unflatten From JSON(JSON string=w204, type and defaults=T17 {"Info"={"Resource"="Zenone", "Problem"=0.0, "Timestamp"=0.0}, "Data"={"Operation_mode"="Grid connected", "solution_feasible"=0.0, "Optimal_slack"="AFE 1", "setpoints"=[], "upper_layer_grid_info"={"Frequency"=0.0, "Angle"=0.0, "Magnitude"=0.0}, "SC_soc"=0.0, "PV"={"perun"=0.0, "solarmax"=0.0, "facade"=0.0, "emul4"=0.0, "emul5"=0.0, "emul6"=0.0, "emul7"=0.0}, "P_pv_facade"=0.0}} ("IN iOPF"), error in (no error)=w205) -> (value=w202:T17, error out=w206:errorcluster)  [unwired: 4 in]
      }
      frame Error {
        n62 = local read "IN cOPF"() -> (w207:T17)
      }
    }
    n63 = local read "Stop"() -> (w198:bool)
    n64 = local write "IN cOPF"(w197) -> ()
  }
  n65 = while {
    tunnel: w82 -> [w220]
    tunnel: w81 -> [w219]
    tunnel: w77 -> [w216]
    tunnel: w76 -> [w215]
    tunnel: [w214] -> w79
    tunnel: [w213] -> w78
    stop <- w212 stop-if-true
    n66 = local read "OUT cOPF"() -> (w217:T17)
    n67 = Flatten To JSON(anything=w217, error in (no error)=w215) -> (JSON string=w218:string, 11:w211:errorcluster)  [unwired: 1 in]
    n68 = UDP Write(address=w219, port or service name=w220, connection ID=w216, data in=w218, 8:w211, 9:50 ("timeout ms (25000)")) -> (error out=w213:errorcluster, 3:w214:refnum<k16>)
    n69 = local read "Stop"() -> (w212:bool)
    n70 = Wait Until Next ms Multiple(millisecond multiple=u32 100) -> ()  [unwired: 1 out]
  }
  n71 = while {
    tunnel: w16 -> [w241]
    tunnel: w15 -> [w240]
    tunnel: [w239] -> w18
    tunnel: [w238] -> w17
    tunnel: 8 ("millisecond multiple") -> [w225]
    shift-right: [w221] -> _
    shift-left: dbl[] [0.0] -> [w226]
    stop <- w243 stop-if-true
    (unwired) i64 0 ("Iteration Duration")
    n72 = Wait Until Next ms Multiple(millisecond multiple=u32 100) -> ()  [unwired: 1 out]
    n73 = UDP Read(connection ID=w241, max size (548)=2000, timeout ms (25000)=50, 8:w240) -> (data out=w242:string, error out=w237:errorcluster, 3:w238:refnum<k16>)  [unwired: 2 out]
    n74 = call <vilib>:"Is Empty.vi"("JSON"=w242) -> ("Empty"=w244:bool)  [unwired: 4 in]
    n75 = Not(x=w244) -> (.not. x?=→"PV data":bool)
    n76 = case shown="No Error" w237 {
      tunnel: w237 -> [w260 w263]
      tunnel: w242 -> [w259 _]
      tunnel: [w261 w263] -> w239
      tunnel: [w258 w262] -> w231
      frame No Error {
        n77 = Unflatten From JSON(JSON string=w259, type and defaults=T7 {"Info"={"Resource"="Zenone", "Problem"=FALSE, "Timestamp"=0.0}, "Data"={"Status 1"=FALSE, "Status 2"=FALSE, "measurements"={"V_PV1"=0.0, "V_CAP1"=0.0, "V_PV2"=0.0, "V_CAP2"=0.0, "V_grid2"=0.0, "V_PV3"=0.0, "V_CAP3"=0.0, "V_grid3"=0.0, "V_PV4"=0.0, "V_CAP4"=0.0, "V_grid4"=0.0, "V_grid1"=0.0, "P1"=0.0, "P2"=0.0, "P3"=0.0, "P4"=0.0}, "Status 3"=FALSE, "Status 4"=FALSE, "measurements SC"={"V_SC"=0.0, "V_CAP"=0.0, "V_grid"=0.0, "P"=0.0, "SOC"=0.0}, "Status SC"=FALSE, "Forming/Following"=FALSE, "Start forming"=FALSE, "SC references"={"Vdc"=0.0, "Pdc"=0.0}, "Start following"=FALSE}} ("PV+SC"), error in (no error)=w260) -> (value=w258:T7, error out=w261:errorcluster)  [unwired: 4 in]
      }
      frame Error {
        n78 = local read "IN PV+SC"() -> (w262:T7)
      }
    }
    n79 = Array Size(array=w226) -> (size(s)=w224:i32)
    n80 = Equal?(x=w224, y=w225) -> (x = y?=w227:bool)
    n81 = Unbundle By Name(w231) -> ("Data.measurements SC.SOC"=w223:dbl)
    n82 = case shown="True" w227 {
      tunnel: [w248 w252] -> w221
      tunnel: w226 -> [w247 w256]
      tunnel: w225 -> [_ w250]
      tunnel: w223 -> [w246 w249]
      frame False {
        n83 = Insert Into Array(array=w247, new element=w246) -> (w248:dbl[])  [unwired: 1 in]
      }
      frame True {
        n84 = Array Subset(array=w256, index=0) -> (w254:dbl[])  [unwired: 1 in]
        n85 = Build Array (concatenate)(w249, w254) -> (w253:dbl[])
        n86 = Delete From Array(array=w253, length=1, index=w250) -> (array with subset deleted=w252:dbl[])  [unwired: 1 out]
      }
    }
    n87 = call-poly <vilib>:"Mean.vi"("X"=w221) -> ("mean"=w222:dbl)  [unwired: 1 out]
    n88 = Select(t=w222, s="Real_SOC", f="SOC") -> (s? t:f=w232:dbl)
    n89 = Bundle By Name(cluster=w231, "Data.measurements SC.SOC"=w232) -> (w234:T7)
    n90 = Bundle("SOC"=w232) -> (→"SOC":cluster{"SOC":dbl})  [unwired: 1 in]
    n91 = local read "Stop"() -> (w243:bool)
    n92 = local write "IN PV+SC"(w234) -> ()
  }
  n93 = while {
    tunnel: w12 -> [w266]
    tunnel: w11 -> [w265]
    tunnel: w7 -> [w271]
    tunnel: w6 -> [w274]
    tunnel: [w267] -> w9
    tunnel: [w268] -> w8
    stop <- w273 stop-if-true
    n94 = local read "OUT PV+SC"() -> (w275:T7)
    n95 = Flatten To JSON(anything=w275, error in (no error)=w274) -> (JSON string=w269:string, 11:w270:errorcluster)  [unwired: 1 in]
    n96 = Wait Until Next ms Multiple(millisecond multiple=u32 100) -> ()  [unwired: 1 out]
    n97 = case shown="True" "Send sp DC?" {
      tunnel: w270 -> [w276 w284]
      tunnel: w269 -> [_ w283]
      tunnel: w271 -> [w277 w282]
      tunnel: [w277 w281] -> w267
      tunnel: [w276 w280] -> w268
      tunnel: w266 -> [_ w279]
      tunnel: w265 -> [_ w278]
      frame False {
      }
      frame True {
        n98 = UDP Write(address=w278, port or service name=w279, connection ID=w282, data in=w283, 8:w284) -> (error out=w280:errorcluster, 3:w281:refnum<k16>)  [unwired: 1 in]
      }
    }
    n99 = local read "Stop"() -> (w273:bool)
  }
  n100 = call-poly <vilib>:"Read Delimited Spreadsheet.vi"("file path (dialog if empty)"=path "C:/Users/admin/Documents/git-clones/acdc_centralized_controller2/Data/Zenone_profile.csv", "format (%.3f)"="%.3f", "delimiter (\\t)"=" " ("delimiter (\\t)")) -> ("all rows"=w98:dbl[][])  [unwired: 7 in, 5 out]
  n101 = Matrix Size(0:w98) -> (1:w90:i32)  [unwired: 1 out]
  n102 = while {
    shift-right: [w297] -> _
    shift-left: 0 ("number of rows") -> [w295]
    tunnel: w98 -> [w290]
    tunnel: w90 -> [w291]
    stop <- w298 stop-if-true
    (unwired) 3.0 ("element")
    (unwired) 6.0 ("element")
    n103 = Quotient & Remainder(x=w295, y=w291) -> (x-y*floor(x/y)=w294:i32)  [unwired: 1 out]
    n104 = Index Array(array=w290, index (row)=w294) -> (element=w288:dbl[])  [unwired: 1 in]
    n105 = Multiply(x=0.36 ("Numeric"), y=w288) -> (x*y=w289:dbl[])
    n106 = Index Array(array=w289) -> (element #1=w286:dbl, element #2=w285:dbl)  [unwired: 2 in]
    n107 = Absolute Value(x=w285) -> (abs(x)=→"Zenone_Q":dbl)
    n108 = Absolute Value(x=w286) -> (abs(x)=→"Zenone_P":dbl)
    n109 = local read "Stop"() -> (w298:bool)
    n110 = Increment(x=w294) -> (x+1=w297:i32)
    n111 = Wait (ms)(milliseconds to wait=u32 1000) -> ()  [unwired: 1 out]
  }
  n112 = node-c288(i64 100 ("Period")) -> (w5:T26)  [unwired: 3 in]
  n113 = timed-loop {
    shift-right: [w319] -> _
    shift-left: w110 -> [w320]
    shift-right: [w317] -> _
    shift-left: w108 -> [w318]
    tunnel: "nb instances" -> [w316]
    shift-right: [w309] -> _
    shift-left: State_Machine."Grid connected" ("State") -> [w310]
    shift-right: [w299] -> _
    shift-left: errorcluster {"status"=FALSE, "code"=0, "source"=""} ("error constant") -> [w300]
    timing: w5 -> [_]
    timing-out: [_] -> w4
    stop <- "Stop" stop-if-true
    # "State Machine While Loop"
    n114 = node-c288() -> ()  [unwired: 1 in, 1 out]
    n115 = case "State Machine Case Structure" shown="\"Prepare for connection\"" w310 {
      tunnel: "IN synchro" -> [w350 w451 w563 w679 w803]
      tunnel: "IN AFE" -> [w349 w452 w564 w680 w802]
      tunnel: "IN cOPF" -> [w348 w453 w565 w681 w801]
      tunnel: "IN iOPF" -> [w347 w454 w566 w682 w800]
      tunnel: w320 -> [w346 w450 w562 w678 w799]
      tunnel: [w346 w449 w562 w678 w799] -> w319
      tunnel: w318 -> [w345 w448 w561 w677 w798]
      tunnel: [w345 w447 w561 w677 w798] -> w317
      tunnel: w316 -> [_ w446 _ _ _]
      tunnel: [w341 w438 w557 w673 w794] -> w315
      tunnel: [w343 w440 w558 w674 w795] -> w314
      tunnel: [w342 w439 w559 w675 w796] -> w313
      tunnel: [w344 w441 w560 w676 w797] -> w312
      tunnel: [w329 w427 w547 w661 w782] -> w309
      tunnel: "IN PV+SC" -> [w335 w431 w551 w666 w787]
      tunnel: [w334 w428 w548 w663 w784] -> w303
      tunnel: "IN Meteo" -> [w328 w424 w545 w659 w778]
      tunnel: "SCADA" -> [_ _ w542 w657 w774]
      tunnel: w300 -> [w325 w420 w537 w653 w769]
      tunnel: [w323 w418 w535 w652 w767] -> w299
      frame "Grid connected", Default {
        # "Grid connected - Display a dialog box with a message specific to State 1, then go back to the Wait for Event state."
        n116 = flat-sequence {
          tunnel: w350 -> [w376]
          tunnel: w349 -> [w377]
          tunnel: w348 -> [w375]
          tunnel: w347 -> [w374]
          tunnel: [w377] -> w340
          tunnel: [w376] -> w339
          tunnel: [w375] -> w338
          tunnel: [w374] -> w337
          tunnel: [w359] -> w336
          tunnel: w335 -> [w367]
          tunnel: [w373] -> w333
          tunnel: [w367] -> w332
          tunnel: [w359] -> w331
          tunnel: w328 -> [w363]
          tunnel: [w362] -> w327
          tunnel: [w360] -> w326
          tunnel: w325 -> [w360]
          tunnel: w340 -> [w411]
          tunnel: w339 -> [w410]
          tunnel: w338 -> [w409]
          tunnel: w337 -> [w408]
          tunnel: w336 -> [w406]
          tunnel: w333 -> [w405]
          tunnel: w332 -> [w403]
          tunnel: w331 -> [w400]
          tunnel: [w415] -> w344
          tunnel: [w414] -> w343
          tunnel: [w413] -> w342
          tunnel: [w412] -> w341
          tunnel: [w404] -> w334
          tunnel: w327 -> [w392]
          tunnel: [w388] -> w324
          tunnel: w326 -> [w388]
          frame #0 {
            # "from island OPF"
            # "from connected OPF"
            # "from resource"
            # "from synchrocheck"
            n117 = Unbundle By Name(w367) -> ("Data.Forming/Following"=→"forming SC?":bool, "Data.measurements SC.SOC"=w364:dbl)
            n118 = Unbundle By Name(w376) -> ("Data.Synchronised?"=→"synchronised?":bool, "Data.V_UpStream"=w366:T23, "Data.V_Downstream"=w365:T23)
            n119 = Unbundle By Name(w363) -> ("Data.PV_mpp"=w362:T31)
            n120 = Unbundle By Name(w377) -> ("Data.Forming/Following"=w382:bool[])
            n121 = Unbundle By Name(w375) -> ("Data.solution_feasible"=w370:dbl, "Data.setpoints"=w357:dbl[])
            n122 = Unbundle By Name(w374) -> ("Data.solution_feasible"=w372:dbl)
            n123 = local write "to connected-island"(FALSE ("to connected island")) -> ()
            n124 = local write "to grid connection"(TRUE ("to grid connection")) -> ()
            n125 = local write "to prepare for island"(FALSE ("to prepare for island")) -> ()
            n126 = local write "to island"(FALSE ("to island")) -> ()
            n127 = local write "to prepare for grid connection"(FALSE ("to prepare for grid connection")) -> ()
            n128 = local read "old_sp_island"() -> (w356:dbl[])
            n129 = local read "old_sp_island_bool"() -> (w358:bool)
            n130 = Not Equal To 0?(x=w370) -> (x != 0?=→"cOPF valid?":bool)
            n131 = Not Equal To 0?(x=w372) -> (x != 0?=→"iOPF valid":bool)
            n132 = local write "setpoints"(w357) -> ()
            n133 = Or Array Elements(Boolean array=w382) -> (logical OR=→"forming AFE?":bool)
            n134 = local write "SC_soc"(w364) -> ()
            n135 = call "up_grid_data.vi"("Data.V_Downstream"=w365, "Data.V_UpStream"=w366) -> ("upper layer grid info"=w373:T30)  [unwired: 5 in, 4 out]
            n136 = Select(t=w356, s=w358, f=w357) -> (s? t:f=w359:dbl[])
          }
          frame #1 {
            # "send to island OPF"
            # "send to resource"
            # "send to connected OPF"
            # "send to synchrocheck"
            n137 = local read "P_pv_facade"() -> (w389:dbl)
            n138 = Get Date/Time In Seconds() -> (seconds since 1Jan1904=w386:timestamp)
            n139 = local read "SC_soc"() -> (w394:dbl)
            n140 = local read "SC_soc"() -> (w393:dbl)
            n141 = call "distribute_setpoints.vi"("setpoints"=w406, "upper layer grid info"=w405) -> ("references"=w407:T16)  [unwired: 9 in]
            n142 = call "distribute_setpoints_DC.vi"("setpoints"=w400) -> ("reference_DC"=w401:T12)  [unwired: 10 in]
            n143 = To Double Precision Float(number=w386) -> (double precision float=w385:dbl)
            n144 = Bundle By Name(cluster=w409, "Data.Operation_mode"="Grid connected" ("Operation_mode"), "Data.upper_layer_grid_info"=w405, "Data.SC_soc"=w394, "Data.P_pv_facade"=w389, "Data.PV"=w392) -> (w413:T17)
            n145 = Bundle By Name(cluster=w408, "Data.Operation_mode"="Grid connected" ("Operation_mode"), "Data.upper_layer_grid_info"=w405, "Data.SC_soc"=w393, "Data.P_pv_facade"=w389, "Data.PV"=w392) -> (w415:T17)
            n146 = Bundle By Name(cluster=w403, "Data.Start following"=TRUE, "Data.Start forming"=FALSE, "Data.SC references"=w401) -> (w404:T7)
            n147 = Bundle By Name(cluster=w410, "Info.Timestamp"=w385, "Data.close/open relay"=TRUE, "Data.Operation mode"="Grid connected" ("Operation_mode")) -> (w412:T20)
            n148 = Bundle By Name(cluster=w411, "Info.Timestamp"=w385, "Data.Start forming 2"=FALSE, "Data.Start following 2"=TRUE, "Data.Start following 1"=TRUE, "Data.Start forming 1"=FALSE, "Data.references"=w407) -> (w414:T13)
            n149 = local write "old_sp_island_bool"(FALSE ("old_sp_island_bool")) -> ()
          }
        }
        n150 = case shown="True" "to prepare for island" {
          tunnel: [State_Machine."Grid connected" ("State") State_Machine."Prepare for island" ("State")] -> w329
          tunnel: [w351 w353] -> w323
          tunnel: w324 -> [w351 w353]
          frame False {
          }
          frame True {
            n151 = local write "Reset_magnitude"(TRUE ("Rest_PI_V")) -> ()
          }
        }
      }
      frame "Prepare for island" {
        n152 = flat-sequence {
          tunnel: w454 -> [w485]
          tunnel: w453 -> [w484]
          tunnel: w452 -> [w482]
          tunnel: w451 -> [w483]
          tunnel: w450 -> [w494]
          tunnel: w448 -> [w492]
          tunnel: w446 -> [w488]
          tunnel: [w493] -> w445
          tunnel: [w491] -> w444
          tunnel: [w490] -> w443
          tunnel: [w489] -> w442
          tunnel: [w485] -> w437
          tunnel: [w484] -> w436
          tunnel: [w483] -> w435
          tunnel: [w482] -> w434
          tunnel: [w474] -> w433
          tunnel: [w481] -> w432
          tunnel: w431 -> [w475]
          tunnel: [w475] -> w430
          tunnel: [w474] -> w429
          tunnel: w424 -> [w466]
          tunnel: [w465] -> w423
          tunnel: [w463] -> w421
          tunnel: w420 -> [w463]
          tunnel: w445 -> [w533]
          tunnel: w444 -> [w532]
          tunnel: w443 -> [w512]
          tunnel: w442 -> [w513]
          tunnel: w437 -> [w523]
          tunnel: w436 -> [w522]
          tunnel: w435 -> [w521]
          tunnel: w434 -> [w520]
          tunnel: w433 -> [w518]
          tunnel: w432 -> [w507]
          tunnel: w430 -> [w517]
          tunnel: w429 -> [w514]
          tunnel: [w533] -> w449
          tunnel: [w532] -> w447
          tunnel: [w527] -> w441
          tunnel: [w526] -> w440
          tunnel: [w525] -> w439
          tunnel: [w524] -> w438
          tunnel: [w516] -> w428
          tunnel: [w513] -> w426
          tunnel: [w512] -> w425
          tunnel: w423 -> [w502]
          tunnel: [w498] -> w419
          tunnel: w421 -> [w498]
          frame #0 {
            # "from island OPF"
            # "from connected OPF"
            # "from resource"
            # "from synchrocheck"
            n153 = Unbundle By Name(w466) -> ("Data.PV_mpp"=w465:T31)
            n154 = Unbundle By Name(w475) -> ("Data.Forming/Following"=w476:bool, "Data.measurements SC.SOC"=w467:dbl)
            n155 = Unbundle By Name(w484) -> ("Data.solution_feasible"=w478:dbl, "Data.setpoints"=w474:dbl[])
            n156 = Unbundle By Name(w482) -> ("Data.Forming/Following"=w495:bool[])
            n157 = Unbundle By Name(w485) -> ("Data.solution_feasible"=w479:dbl)
            n158 = Unbundle By Name(w483) -> ("Data.Synchronised?"=w487:bool, "Data.V_UpStream"=w469:T23, "Data.V_Downstream"=w468:T23)
            n159 = local write "to connected-island"(FALSE ("to connected island")) -> ()
            n160 = local write "to grid connection"(FALSE ("to grid connection")) -> ()
            n161 = local write "to prepare for island"(TRUE ("to prepare for island")) -> ()
            n162 = local write "to island"(FALSE ("to island")) -> ()
            n163 = local write "to prepare for grid connection"(FALSE ("to prepare for grid connection")) -> ()
            n164 = local write "synchronised?"(w487) -> ()
            n165 = Or Array Elements(Boolean array=w495) -> (logical OR=w486:bool)
            n166 = local write "setpoints"(w474) -> ()
            n167 = local write "forming SC?"(w476) -> ()
            n168 = local write "SC_soc"(w467) -> ()
            n169 = Not Equal To 0?(x=w478) -> (x != 0?=w477:bool)
            n170 = Not Equal To 0?(x=w479) -> (x != 0?=w480:bool)
            n171 = local write "forming AFE?"(w486) -> ()
            n172 = call "check multiple instances.vi"("nb instances"=w488, "array elements in"=w494, "new element"=w477) -> ("array elements out"=w493:bool[], "out"=w489:bool)  [unwired: 7 in]
            n173 = local write "cOPF valid?"(w477) -> ()
            n174 = call "check multiple instances.vi"("nb instances"=w488, "array elements in"=w492, "new element"=w480) -> ("array elements out"=w491:bool[], "out"=w490:bool)  [unwired: 7 in]
            n175 = local write "iOPF valid"(w480) -> ()
            n176 = call "up_grid_data.vi"("Data.V_Downstream"=w468, "Data.V_UpStream"=w469) -> ("upper layer grid info"=w481:T30)  [unwired: 5 in, 4 out]
          }
          frame #1 {
            # "send to island OPF"
            # "send to resource"
            # "send to connected OPF"
            # "send to synchrocheck"
            n177 = Get Date/Time In Seconds() -> (seconds since 1Jan1904=w497:timestamp)
            n178 = local read "P_pv_facade"() -> (w499:dbl)
            n179 = local read "optimal_slack"() -> (w530:string)
            n180 = local read "optimal_slack"() -> (w531:string)
            n181 = To Double Precision Float(number=w497) -> (double precision float=w496:dbl)
            n182 = call "distribute_setpoints_DC.vi"("setpoints"=w514) -> ("reference_DC"=w506:T12)  [unwired: 10 in]
            n183 = call "distribute_setpoints.vi"("setpoints"=w518, "upper layer grid info"=w507) -> ("references"=w519:T16)  [unwired: 9 in]
            n184 = local read "SC_soc"() -> (w504:dbl)
            n185 = local read "SC_soc"() -> (w503:dbl)
            n186 = Bundle By Name(cluster=w522, "Data.Operation_mode"="Prepare Island" ("Operation_mode"), "Data.Optimal_slack"=w530, "Data.upper_layer_grid_info"=w507, "Data.SC_soc"=w504, "Data.P_pv_facade"=w499, "Data.PV"=w502) -> (w525:T17)
            n187 = Bundle By Name(cluster=w523, "Data.Operation_mode"="Prepare Island" ("Operation_mode"), "Data.Optimal_slack"=w531, "Data.upper_layer_grid_info"=w507, "Data.SC_soc"=w503, "Data.P_pv_facade"=w499, "Data.PV"=w502) -> (w527:T17)
            n188 = Bundle By Name(cluster=w521, "Info.Timestamp"=w496, "Data.close/open relay"=TRUE, "Data.Operation mode"="Prepare Island" ("Operation_mode")) -> (w524:T20)
            n189 = Bundle By Name(cluster=w520, "Info.Timestamp"=w496, "Data.Start forming 2"=FALSE, "Data.Start following 2"=TRUE, "Data.Start following 1"=TRUE, "Data.Start forming 1"=FALSE, "Data.references"=w519) -> (w526:T13)
            n190 = Bundle By Name(cluster=w517, "Data.Start following"=TRUE, "Data.Start forming"=FALSE, "Data.SC references"=w506) -> (w516:T7)
          }
        }
        n191 = disable-structure shown="Disabled" {
          disable-tunnel: [w458 _] -> _
          disable-tunnel: "to connected-island" -> [w457 _]
          disable-tunnel: w426 -> [w456 _]
          disable-tunnel: w425 -> [w455 _]
          frame Disabled {
            n192 = Compound Arithmetic op=AND(w456, w455, w457) -> (w458:bool)
          }
          frame Enabled {
          }
        }
        n193 = case shown="False" "to connected-island" {
          tunnel: [State_Machine."Prepare for island" ("State") State_Machine."Forming but connected" ("State")] -> w427
          tunnel: [w459 w461] -> w418
          tunnel: w419 -> [w459 w461]
          frame False {
          }
          frame True {
            # "only go to next state if OPFs are feasible for 7 timesteps"
          }
        }
      }
      frame "Forming but connected" {
        # "Island - Display a dialog box with a message specific to State 3, then go back to the Wait for Event state."
        n194 = flat-sequence {
          tunnel: w566 -> [w602]
          tunnel: w565 -> [w601]
          tunnel: w564 -> [w577]
          tunnel: w563 -> [w600]
          tunnel: [w602] -> w556
          tunnel: [w601] -> w555
          tunnel: [w600] -> w554
          tunnel: [w580] -> w553
          tunnel: [w585] -> w552
          tunnel: w551 -> [w594]
          tunnel: [w594] -> w550
          tunnel: [w580] -> w549
          tunnel: [w591] -> w546
          tunnel: w545 -> [w589]
          tunnel: [w588] -> w544
          tunnel: w542 -> [w586]
          tunnel: [w584] -> w541
          tunnel: [w581] -> w540
          tunnel: ["Reset_magnitude"] -> w539
          tunnel: [w578] -> w538
          tunnel: w537 -> [w578]
          tunnel: [w577] -> w534
          tunnel: w556 -> [w628]
          tunnel: w555 -> [w643]
          tunnel: w554 -> [w642]
          tunnel: w553 -> [w640]
          tunnel: w552 -> [w623]
          tunnel: w550 -> [w639]
          tunnel: w549 -> [w636]
          tunnel: [w647] -> w560
          tunnel: [w646] -> w559
          tunnel: [w645] -> w558
          tunnel: [w644] -> w557
          tunnel: [w638] -> w548
          tunnel: w546 -> [_]
          tunnel: w544 -> [w627]
          tunnel: w541 -> [w610]
          tunnel: w540 -> [w611]
          tunnel: w539 -> [w617]
          tunnel: [w613] -> w536
          tunnel: w538 -> [w613]
          tunnel: w534 -> [w612]
          frame #0 {
            # "from island OPF"
            # "from connected OPF"
            # "from resource"
            # "from synchrocheck"
            n195 = Unbundle By Name(w594) -> ("Data.Forming/Following"=w595:bool, "Data.measurements SC.SOC"=w590:dbl)
            n196 = Unbundle By Name(w602) -> ("Data.solution_feasible"=w599:dbl, "Data.upper_layer_grid_info"=w591:T30)  [unwired: 1 out]
            n197 = Unbundle By Name(w577) -> ("Data.Forming/Following"=w609:bool[])
            n198 = Unbundle By Name(w601) -> ("Data.solution_feasible"=w598:dbl, "Data.setpoints"=w580:dbl[])
            n199 = Unbundle By Name(w600) -> ("Data.Synchronised?"=w604:bool, "Data.V_UpStream"=w593:T23, "Data.V_Downstream"=w592:T23)
            n200 = Unbundle By Name(w586) -> ("Data.Voltage mag"=w583:dbl[])
            n201 = Unbundle By Name(w589) -> ("Data.PV_mpp"=w588:T31)
            n202 = local write "to connected-island"(TRUE ("to prepare for grid connection")) -> ()
            n203 = local write "to prepare for grid connection"(FALSE ("to prepare for grid connection")) -> ()
            n204 = local write "to grid connection"(FALSE ("to grid connection")) -> ()
            n205 = local write "to prepare for island"(FALSE ("to prepare for island")) -> ()
            n206 = local write "to island"(FALSE ("to island")) -> ()
            n207 = local write "synchronised?"(w604) -> ()
            n208 = Not Equal To 0?(x=w598) -> (x != 0?=w597:bool)
            n209 = local write "setpoints"(w580) -> ()
            n210 = Not Equal To 0?(x=w599) -> (x != 0?=w596:bool)
            n211 = Or Array Elements(Boolean array=w609) -> (logical OR=w603:bool)
            n212 = local write "forming SC?"(w595) -> ()
            n213 = Index Array(array=w583, index=18) -> (element=w581:dbl)
            n214 = local write "SC_soc"(w590) -> ()
            n215 = local write "forming AFE?"(w603) -> ()
            n216 = local write "cOPF valid?"(w597) -> ()
            n217 = call "up_grid_data.vi"("Data.V_Downstream"=w592, "Data.V_UpStream"=w593) -> ("upper layer grid info"=w585:T30)  [unwired: 5 in, 4 out]
            n218 = local write "iOPF valid"(w596) -> ()
            n219 = Unbundle By Name(w585) -> ("Magnitude"=w584:dbl)
          }
          frame #1 {
            # "!!! NO PID !!!"
            # "send to island OPF"
            # "send to connected OPF"
            # "send to resource"
            # "send to synchrocheck"
            n220 = call <userlib>:"Boolean Trigger__ogtk.vi"("Boolean Input"=w617) -> ("Rising Edge"=w616:bool)  [unwired: 1 in, 1 out]
            n221 = call "PID2_2V.vi"("reinitialize? (F)"=w616, "V_afe"=w611, "V_up"=w610) -> ()  [unwired: 8 in, 1 out]
            n222 = Unbundle(w623) -> ("Frequency"=w621:dbl)  [unwired: 2 out]
            "V_freq" <- w621
            n223 = local read "optimal_slack"() -> (w651:string)
            n224 = local read "P_pv_facade"() -> (w624:dbl)
            n225 = local read "optimal_slack"() -> (w650:string)
            n226 = call "distribute_setpoints_DC.vi"("setpoints"=w636) -> ("reference_DC"=w632:T12)  [unwired: 10 in]
            n227 = local read "SC_soc"() -> (w629:dbl)
            n228 = local read "SC_soc"() -> (w630:dbl)
            n229 = Bundle(cluster=T30 {"Frequency"=0.0, "Angle"=0.0, "Magnitude"=0.0} ("upper layer grid info"), "Frequency"=w621, "Angle"=0.0, "Magnitude"=w610) -> (w635:T30)
            n230 = Bundle("Magnitude"=w610) -> (→"V control":cluster{"Magnitude":dbl})  [unwired: 1 in]
            n231 = call "distribute_setpoints.vi"("setpoints"=w640, "upper layer grid info"=w635) -> ("references"=w641:T16)  [unwired: 9 in]
            n232 = Bundle By Name(cluster=w643, "Data.Operation_mode"=T29 "Forming but connected" ("Operation_mode"), "Data.Optimal_slack"=w650, "Data.upper_layer_grid_info"=w623, "Data.SC_soc"=w630, "Data.P_pv_facade"=w624, "Data.PV"=w627) -> (w646:T17)
            n233 = Bundle By Name(cluster=w628, "Data.Operation_mode"=T29 "Forming but connected" ("Operation_mode"), "Data.Optimal_slack"=w651, "Data.upper_layer_grid_info"=w623, "Data.SC_soc"=w629, "Data.P_pv_facade"=w624, "Data.PV"=w627) -> (w647:T17)
            n234 = Bundle By Name(cluster=w639, "Data.Start following"=FALSE, "Data.Start forming"=TRUE, "Data.SC references"=w632) -> (w638:T7)
            n235 = Bundle By Name(cluster=w642, "Data.close/open relay"=TRUE, "Data.Operation mode"=T29 "Forming but connected" ("Operation_mode")) -> (w644:T20)
            n236 = Bundle By Name(cluster=w612, "Data.Start forming 2"=FALSE, "Data.Start following 2"=TRUE, "Data.Start following 1"=FALSE, "Data.Start forming 1"=TRUE, "Data.references"=w641) -> (w645:T13)
            n237 = local write "Reset_magnitude"(FALSE ("Rest_PI_V")) -> ()
            "V_upstream" <- w610
            "V_afe" <- w611
            "V_control" <- w610
          }
        }
        n238 = case shown="True" "to island" {
          tunnel: [State_Machine."Forming but connected" ("State") State_Machine."Island" ("State")] -> w547
          tunnel: w536 -> [w567 w572]
          tunnel: [w567 w572] -> w535
          frame False {
          }
          frame True {
            # "only go to next state if OPFs are feasible\n for 7 timesteps"
            n239 = local read "V_control"() -> (w573:dbl)
            n240 = local read "V_freq"() -> (→"V_freq_for_island":dbl)
            n241 = local write "Reset_magnitude"(TRUE ("Rest_PI_V")) -> ()
            n242 = local write "delta angle"(0.0 ("delta angle")) -> ()
            n243 = Add(x=w573, y=0.0) -> (x+y=→"V_control_fix_for_island":dbl)
          }
        }
      }
      frame "Island" {
        # "Island - Display a dialog box with a message specific to State 3, then go back to the Wait for Event state."
        n244 = flat-sequence {
          tunnel: w682 -> [w715]
          tunnel: w681 -> [w714]
          tunnel: w680 -> [w713]
          tunnel: w679 -> [w712]
          tunnel: [w715] -> w672
          tunnel: [w714] -> w671
          tunnel: [w713] -> w670
          tunnel: [w712] -> w669
          tunnel: [w705] -> w668
          tunnel: [w696] -> w667
          tunnel: w666 -> [w706]
          tunnel: [w706] -> w665
          tunnel: [w705] -> w664
          tunnel: [w702] -> w660
          tunnel: w659 -> [w700]
          tunnel: [w699] -> w658
          tunnel: w657 -> [w697]
          tunnel: [w695] -> w656
          tunnel: [w691] -> w655
          tunnel: [w690] -> w654
          tunnel: w672 -> [w736]
          tunnel: w671 -> [w755]
          tunnel: w670 -> [w754]
          tunnel: w669 -> [w753]
          tunnel: w668 -> [w751]
          tunnel: w667 -> [w730]
          tunnel: w665 -> [w750]
          tunnel: w664 -> [w747]
          tunnel: [w759] -> w676
          tunnel: [w758] -> w675
          tunnel: [w757] -> w674
          tunnel: [w756] -> w673
          tunnel: [w749] -> w663
          tunnel: w660 -> [_]
          tunnel: w658 -> [w735]
          tunnel: w656 -> [w728]
          tunnel: w655 -> [w727]
          tunnel: w654 -> [w729]
          frame #0 {
            # "from island OPF"
            # "from connected OPF"
            # "from resource"
            # "from synchrocheck"
            n245 = Unbundle By Name(w706) -> ("Data.Forming/Following"=w707:bool, "Data.measurements SC.SOC"=w701:dbl)
            n246 = Unbundle By Name(w715) -> ("Data.solution_feasible"=w711:dbl, "Data.setpoints"=w705:dbl[], "Data.upper_layer_grid_info"=w702:T30)
            n247 = Unbundle By Name(w713) -> ("Data.Forming/Following"=w722:bool[])
            n248 = Unbundle By Name(w714) -> ("Data.solution_feasible"=w710:dbl)
            n249 = Unbundle By Name(w712) -> ("Data.Synchronised?"=w717:bool, "Data.V_UpStream"=w704:T23, "Data.V_Downstream"=w703:T23)
            n250 = Unbundle By Name(w697) -> ("Data.Voltage mag"=w694:dbl[])  [unwired: 1 out]
            n251 = Unbundle By Name(w700) -> ("Data.PV_mpp"=w699:T31)
            n252 = local write "to connected-island"(FALSE ("to connected island")) -> ()
            n253 = local write "to grid connection"(FALSE ("to grid connection")) -> ()
            n254 = local write "to prepare for island"(FALSE ("to prepare for island")) -> ()
            n255 = local write "to island"(TRUE ("to island")) -> ()
            n256 = local write "to prepare for grid connection"(FALSE ("to prepare for grid connection")) -> ()
            n257 = local write "synchronised?"(w717) -> ()
            n258 = Not Equal To 0?(x=w710) -> (x != 0?=w709:bool)
            n259 = local write "setpoints"(w705) -> ()
            n260 = Not Equal To 0?(x=w711) -> (x != 0?=w708:bool)
            n261 = Or Array Elements(Boolean array=w722) -> (logical OR=w716:bool)
            n262 = local write "forming SC?"(w707) -> ()
            n263 = Index Array(array=w694, index #1=14 ("index"), index #2=18 ("index")) -> (element #2=w691:dbl)  [unwired: 1 out]
            n264 = local write "SC_soc"(w701) -> ()
            n265 = local write "forming AFE?"(w716) -> ()
            n266 = local write "cOPF valid?"(w709) -> ()
            n267 = local write "iOPF valid"(w708) -> ()
            n268 = local read "Reset_magnitude"() -> (w690:bool)
            n269 = call "up_grid_data.vi"("Data.V_Downstream"=w703, "Data.V_UpStream"=w704) -> ("upper layer grid info"=w696:T30)  [unwired: 5 in, 4 out]
            n270 = Unbundle By Name(w696) -> ("Magnitude"=w695:dbl)
          }
          frame #1 {
            (unwired) 230.0 ("Magnitude")
            # "send to island OPF"
            # "send to connected OPF"
            # "send to resource"
            # "send to synchrocheck"
            n271 = local read "V_control_fix_for_island"() -> (w724:dbl)
            n272 = Unbundle(w730) -> ()  [unwired: 3 out]
            n273 = call <userlib>:"Boolean Trigger__ogtk.vi"("Boolean Input"=w729) -> ()  [unwired: 1 in, 2 out]
            n274 = local read "optimal_slack"() -> (w763:string)
            n275 = local read "P_pv_facade"() -> (w731:dbl)
            n276 = local read "optimal_slack"() -> (w762:string)
            n277 = call "PID2_2V.vi"("V_afe"=w727, "V_up"=w728) -> ()  [unwired: 9 in, 1 out]
            n278 = call "distribute_setpoints_DC.vi"("setpoints"=w747) -> ("reference_DC"=w740:T12)  [unwired: 10 in]
            n279 = Bundle(cluster=T30 {"Frequency"=0.0, "Angle"=0.0, "Magnitude"=0.0} ("upper layer grid info"), "Frequency"=50.0, "Angle"=0.0, "Magnitude"=w724) -> (w743:T30)
            n280 = local read "SC_soc"() -> (w737:dbl)
            n281 = local read "SC_soc"() -> (w738:dbl)
            n282 = call "distribute_setpoints.vi"("setpoints"=w751, "upper layer grid info"=w743) -> ("references"=w752:T16)  [unwired: 9 in]
            n283 = local write "V_upstream"(w728) -> ()
            n284 = local write "V_afe"(w727) -> ()
            n285 = Bundle("V_control_fix_for_island"=w724) -> (w726:cluster{"V_control_fix_for_island":dbl})  [unwired: 1 in]
            n286 = Bundle By Name(cluster=w755, "Data.Operation_mode"="Island" ("Operation_mode"), "Data.Optimal_slack"=w762, "Data.upper_layer_grid_info"=w730, "Data.SC_soc"=w738, "Data.P_pv_facade"=w731, "Data.PV"=w735) -> (w758:T17)
            n287 = Bundle By Name(cluster=w736, "Data.Operation_mode"="Island" ("Operation_mode"), "Data.Optimal_slack"=w763, "Data.upper_layer_grid_info"=w730, "Data.SC_soc"=w737, "Data.P_pv_facade"=w731, "Data.PV"=w735) -> (w759:T17)
            n288 = Bundle By Name(cluster=w750, "Data.Start following"=FALSE, "Data.Start forming"=TRUE, "Data.SC references"=w740) -> (w749:T7)
            n289 = Bundle By Name(cluster=w753, "Data.close/open relay"=FALSE, "Data.Operation mode"="Island" ("Operation_mode")) -> (w756:T20)
            n290 = local write "V control"(w726) -> ()
            n291 = Bundle By Name(cluster=w754, "Data.Start forming 2"=FALSE, "Data.Start following 2"=TRUE, "Data.Start following 1"=FALSE, "Data.Start forming 1"=TRUE, "Data.references"=w752) -> (w757:T13)
            n292 = local write "Reset_magnitude"(FALSE ("Rest_PI_V")) -> ()
          }
        }
        n293 = case shown="True" "to prepare for grid connection" {
          tunnel: [State_Machine."Island" ("State") State_Machine."Prepare for connection" ("State")] -> w661
          tunnel: w653 -> [w683 w686]
          tunnel: [w683 w686] -> w652
          frame False {
          }
          frame True {
            # "only go to next state if OPFs are feasible\n for 7 timesteps"
            n294 = local write "Reset_angle"(TRUE ("Reset_angle")) -> ()
            n295 = local write "delta angle"(0.0 ("delta angle")) -> ()
            n296 = local write "Reset_magnitude"(TRUE ("Rest_PI_V")) -> ()
          }
        }
      }
      frame "Prepare for connection" {
        # "prepare for connection - Display a dialog box with a message specific to State 3, then go back to the Wait for Event state."
        n297 = flat-sequence {
          tunnel: w803 -> [w835]
          tunnel: w802 -> [w836]
          tunnel: w801 -> [w837]
          tunnel: w800 -> [w838]
          tunnel: [w838] -> w793
          tunnel: [w837] -> w792
          tunnel: [w836] -> w791
          tunnel: [w835] -> w790
          tunnel: [w811] -> w789
          tunnel: [w816] -> w788
          tunnel: w787 -> [w829]
          tunnel: [w829] -> w786
          tunnel: [w811] -> w785
          tunnel: [w826] -> w781
          tunnel: [w821] -> w780
          tunnel: [w822] -> w779
          tunnel: w778 -> [w824]
          tunnel: [w823] -> w777
          tunnel: w774 -> [w819]
          tunnel: [w818] -> w773
          tunnel: [w814] -> w772
          tunnel: [w817] -> w771
          tunnel: [w813] -> w770
          tunnel: w769 -> [w813]
          tunnel: ["Reset_angle"] -> w766
          tunnel: [w811] -> w764
          tunnel: w793 -> [w886]
          tunnel: w792 -> [w885]
          tunnel: w791 -> [w884]
          tunnel: w790 -> [w883]
          tunnel: w789 -> [w881]
          tunnel: w788 -> [w870]
          tunnel: w786 -> [w880]
          tunnel: w785 -> [w876]
          tunnel: [w890] -> w797
          tunnel: [w889] -> w796
          tunnel: [w888] -> w795
          tunnel: [w887] -> w794
          tunnel: [w879] -> w784
          tunnel: w781 -> [_]
          tunnel: w780 -> [w865]
          tunnel: w779 -> [w864]
          tunnel: w777 -> [w861]
          tunnel: w773 -> [w846]
          tunnel: w772 -> [w847]
          tunnel: w771 -> [w856]
          tunnel: [w853] -> w768
          tunnel: w770 -> [w853]
          tunnel: w766 -> [w852]
          tunnel: [w848] -> w765
          tunnel: w764 -> [w848]
          frame #0 {
            # "from island OPF"
            # "from connected OPF"
            # "from resource"
            # "from synchrocheck"
            n298 = Unbundle By Name(w819) -> ("Data.Voltage mag"=w820:dbl[])  [unwired: 1 out]
            n299 = Unbundle By Name(w824) -> ("Data.PV_mpp"=w823:T31)
            n300 = Unbundle By Name(w829) -> ("Data.Forming/Following"=w830:bool, "Data.measurements SC.SOC"=w825:dbl)
            n301 = Unbundle By Name(w838) -> ("Data.solution_feasible"=w834:dbl, "Data.setpoints"=w811:dbl[], "Data.upper_layer_grid_info"=w826:T30)
            n302 = Unbundle By Name(w836) -> ("Data.Forming/Following"=w845:bool[])
            n303 = Unbundle By Name(w835) -> ("Data.Synchronised?"=w840:bool, "Data.V_UpStream"=w828:T23, "Data.V_Downstream"=w827:T23)
            n304 = Unbundle By Name(w837) -> ("Data.solution_feasible"=w832:dbl)  [unwired: 1 out]
            n305 = local write "to grid connection"(FALSE ("to grid connection")) -> ()
            n306 = local write "to prepare for island"(FALSE ("to prepare for island")) -> ()
            n307 = local write "to island"(FALSE ("to island")) -> ()
            n308 = local write "to prepare for grid connection"(TRUE ("to prepare for grid connection")) -> ()
            n309 = Index Array(array=w820, index=0) -> (element=w814:dbl)
            n310 = Not Equal To 0?(x=w832) -> (x != 0?=w831:bool)
            n311 = Not Equal To 0?(x=w834) -> (x != 0?=w833:bool)
            n312 = local write "synchronised?"(w840) -> ()
            n313 = local read "Reset_magnitude"() -> (w817:bool)
            n314 = Or Array Elements(Boolean array=w845) -> (logical OR=w839:bool)
            n315 = local write "forming SC?"(w830) -> ()
            n316 = local write "setpoints"(w811) -> ()
            n317 = local write "SC_soc"(w825) -> ()
            n318 = local write "cOPF valid?"(w831) -> ()
            n319 = local write "iOPF valid"(w833) -> ()
            n320 = local write "forming AFE?"(w839) -> ()
            n321 = call "up_grid_data_prepareConnection.vi"("Data.V_Downstream"=w827, "Data.V_UpStream"=w828) -> ("upper layer grid info"=w816:T30, "DOWN_Angle_unwrap"=w822:dbl, "UP_Angle_unwrap"=w821:dbl)  [unwired: 5 in, 2 out]
            n322 = Unbundle By Name(w816) -> ("Magnitude"=w818:dbl)
          }
          frame #1 {
            # "reduce K_p, so we don't have a step"
            # "send to island OPF"
            # "send to connected OPF"
            # "send to resource"
            # "send to synchrocheck"
            n323 = Subtract(x=w865, y=w864) -> (x-y=w850:dbl)
            "delta angle" <- w850
            n324 = Unbundle(w870) -> ()  [unwired: 3 out]
            n325 = call "PID2.vi"("Rest_PI_theta"=w852, "input"=w864, "setpoint"=w865) -> ("output"=w867:dbl)  [unwired: 8 in]
            n326 = call <userlib>:"Boolean Trigger__ogtk.vi"("Boolean Input"=w856) -> ("Rising Edge"=w857:bool)  [unwired: 1 in, 1 out]
            n327 = local read "P_pv_facade"() -> (w858:dbl)
            n328 = local read "optimal_slack"() -> (w893:string)
            n329 = local read "optimal_slack"() -> (w894:string)
            n330 = call "PID2_2V.vi"("reinitialize? (F)"=w857, "V_afe"=w847, "V_up"=w846) -> ()  [unwired: 8 in, 1 out]
            n331 = local read "SC_soc"() -> (w862:dbl)
            n332 = Bundle(cluster=T30 {"Frequency"=0.0, "Angle"=0.0, "Magnitude"=0.0} ("upper layer grid info"), "Frequency"=w867, "Angle"=0.0, "Magnitude"=w846) -> (w871:T30)
            n333 = local read "SC_soc"() -> (w863:dbl)
            n334 = call "distribute_setpoints_DC.vi"("setpoints"=w876) -> ("reference_DC"=w877:T12)  [unwired: 10 in]
            n335 = Bundle(w850) -> (→"V angle":cluster{dbl})  [unwired: 1 in]
            n336 = call "distribute_setpoints.vi"("setpoints"=w881, "upper layer grid info"=w871) -> ("references"=w882:T16)  [unwired: 9 in]
            n337 = local write "V_upstream"(w846) -> ()
            n338 = local write "V_afe"(w847) -> ()
            n339 = Bundle By Name(cluster=w885, "Data.Operation_mode"="Prepare for connection" ("Operation_mode"), "Data.Optimal_slack"=w893, "Data.upper_layer_grid_info"=w870, "Data.SC_soc"=w862, "Data.P_pv_facade"=w858, "Data.PV"=w861) -> (w889:T17)
            n340 = Bundle By Name(cluster=w886, "Data.Operation_mode"="Prepare for connection" ("Operation_mode"), "Data.Optimal_slack"=w894, "Data.upper_layer_grid_info"=w870, "Data.SC_soc"=w863, "Data.P_pv_facade"=w858, "Data.PV"=w861) -> (w890:T17)
            n341 = Bundle("Magnitude"=w846) -> (w855:cluster{"Magnitude":dbl})  [unwired: 1 in]
            n342 = Bundle By Name(cluster=w880, "Data.Start following"=FALSE, "Data.Start forming"=TRUE, "Data.SC references"=w877) -> (w879:T7)
            n343 = Bundle By Name(cluster=w883, "Data.close/open relay"=FALSE, "Data.Operation mode"="Prepare for connection" ("Operation_mode")) -> (w887:T20)
            n344 = local write "V_control"(w846) -> ()
            n345 = Bundle By Name(cluster=w884, "Data.Start forming 2"=FALSE, "Data.Start following 2"=TRUE, "Data.Start following 1"=FALSE, "Data.Start forming 1"=TRUE, "Data.references"=w882) -> (w888:T13)
            n346 = local write "Reset_angle"(FALSE ("Reset_angle")) -> ()
            n347 = local write "Reset_magnitude"(FALSE ("Rest_PI_V")) -> ()
            n348 = local write "V control"(w855) -> ()
          }
        }
        n349 = local read "synchronised?"() -> (w775:bool)
        n350 = And(x="to grid connection", y=w775) -> (x .and. y?=w776:bool)
        n351 = case shown="True" w776 {
          tunnel: [State_Machine."Prepare for connection" ("State") State_Machine."Grid connected" ("State")] -> w782
          tunnel: w768 -> [w804 w808]
          tunnel: [w804 w808] -> w767
          tunnel: w765 -> [_ w807]
          frame False {
          }
          frame True {
            # "only go to next state if OPFs are feasible\n for 7 timesteps"
            n352 = local write "Reset_magnitude"(TRUE ("Rest_PI_V")) -> ()
            "old_sp_island" <- w807
            "old_sp_island_bool" <- TRUE ("Data.Start forming 1")
          }
        }
      }
    }
    "OUT Synchro" <- w315
    "OUT AFE" <- w314
    "OUT cOPF" <- w313
    "OUT iOPF" <- w312
    "OUT PV+SC" <- w303
    n353 = node-c288() -> ()  [unwired: 1 in, 1 out]
  }
  n354 = UDP Close(connection ID=w22, 8:w21) -> ()  [unwired: 2 out]
  n355 = UDP Close(connection ID=w79, 8:w78) -> ()  [unwired: 2 out]
  n356 = UDP Close(connection ID=w9, 8:w8) -> ()  [unwired: 2 out]
  n357 = UDP Close(connection ID=w91, 8:w92) -> ()  [unwired: 2 out]
  n358 = UDP Close(connection ID=w30, 8:w31) -> ()  [unwired: 2 out]
  n359 = UDP Close(connection ID=w48, 8:w49) -> ()  [unwired: 2 out]
  n360 = UDP Close(connection ID=w87, 8:w88) -> ()  [unwired: 2 out]
  n361 = UDP Open(11:w33) -> (port=w42:refnum<k16>, 0:w41:errorcluster)  [unwired: 4 in, 1 out]
  n362 = UDP Open(11:w35) -> (port=w37:refnum<k16>, 0:w36:errorcluster)  [unwired: 4 in, 1 out]
  n363 = String To IP(1:w34) -> (0:w40:u32)
  n364 = UDP Open(11:w58) -> (port=w60:refnum<k16>, 0:w59:errorcluster)  [unwired: 4 in, 1 out]
  n365 = UDP Open(11:w66) -> (port=w73:refnum<k16>, 0:w72:errorcluster)  [unwired: 4 in, 1 out]
  n366 = UDP Open(11:w54) -> (port=w51:refnum<k16>, 0:w50:errorcluster)  [unwired: 4 in, 1 out]
  n367 = UDP Open(11:w65) -> (port=w68:refnum<k16>, 0:w67:errorcluster)  [unwired: 4 in, 1 out]
  n368 = String To IP(1:w57) -> (0:w55:u32)
  n369 = String To IP(1:w64) -> (0:w71:u32)
  n370 = while {
    tunnel: w42 -> [w902]
    tunnel: w41 -> [w901]
    tunnel: [w900] -> w44
    tunnel: [w899] -> w43
    stop <- w905 stop-if-true
    (unwired) i64 0 ("Iteration Duration")
    n371 = Wait Until Next ms Multiple(millisecond multiple=u32 100) -> ()  [unwired: 1 out]
    n372 = UDP Read(connection ID=w902, max size (548)=2000, timeout ms (25000)=50, 8:w901) -> (data out=w903:string, error out=w898:errorcluster, 3:w899:refnum<k16>)  [unwired: 2 out]
    n373 = call <vilib>:"Is Empty.vi"("JSON"=w903) -> ("Empty"=w906:bool)  [unwired: 4 in]
    n374 = Not(x=w906) -> (.not. x?=→"synchro data":bool)
    n375 = case shown="No Error" w898 {
      tunnel: w898 -> [w911 w914]
      tunnel: w903 -> [w910 _]
      tunnel: [w912 w914] -> w900
      tunnel: [w909 w913] -> w904
      frame No Error {
        n376 = Unflatten From JSON(JSON string=w910, type and defaults=T20 {"Info"={"Resource"="SyncroCheck", "Problem"=FALSE, "Timestamp"=0.0}, "Data"={"close/open relay"=TRUE, "Operation mode"="Grid connected", "V_Downstream"={"Phase A"={"Frequency"=0.0, "Magnitude"=0.0, "Angle [Deg]"=0.0}, "Phase B"={"Frequency"=0.0, "Magnitude"=0.0, "Angle [Deg]"=0.0}, "Phase C"={"Frequency"=0.0, "Magnitude"=0.0, "Angle [Deg]"=0.0}, "Phase N"={"Frequency"=0.0, "Magnitude"=0.0, "Angle [Deg]"=0.0}}, "V_UpStream"={"Phase A"={"Frequency"=0.0, "Magnitude"=0.0, "Angle [Deg]"=0.0}, "Phase B"={"Frequency"=0.0, "Magnitude"=0.0, "Angle [Deg]"=0.0}, "Phase C"={"Frequency"=0.0, "Magnitude"=0.0, "Angle [Deg]"=0.0}, "Phase N"={"Frequency"=0.0, "Magnitude"=0.0, "Angle [Deg]"=0.0}}, "Synchronised?"=TRUE}} ("IN synchro"), error in (no error)=w911) -> (value=w909:T20, error out=w912:errorcluster)  [unwired: 4 in]
      }
      frame Error {
        n377 = local read "IN synchro"() -> (w913:T20)
      }
    }
    n378 = local read "Stop"() -> (w905:bool)
    n379 = local write "IN synchro"(w904) -> ()
  }
  n380 = while {
    tunnel: w32 -> [w926]
    tunnel: w40 -> [w925]
    tunnel: w37 -> [w922]
    tunnel: w36 -> [w921]
    tunnel: [w920] -> w39
    tunnel: [w919] -> w38
    stop <- w918 stop-if-true
    n381 = local read "OUT Synchro"() -> (w923:T20)
    n382 = Flatten To JSON(anything=w923, error in (no error)=w921) -> (JSON string=w924:string, 11:w917:errorcluster)  [unwired: 1 in]
    n383 = UDP Write(address=w925, port or service name=w926, connection ID=w922, data in=w924, 8:w917, 9:50 ("timeout ms (25000)")) -> (error out=w919:errorcluster, 3:w920:refnum<k16>)
    n384 = local read "Stop"() -> (w918:bool)
    n385 = Wait Until Next ms Multiple(millisecond multiple=u32 100) -> ()  [unwired: 1 out]
  }
  n386 = while {
    tunnel: w60 -> [w933]
    tunnel: w59 -> [w932]
    tunnel: [w931] -> w62
    tunnel: [w930] -> w61
    stop <- w935 stop-if-true
    (unwired) i64 0 ("Iteration Duration")
    n387 = local read "Stop"() -> (w935:bool)
    n388 = UDP Read(connection ID=w933, max size (548)=2000, timeout ms (25000)=50, 8:w932) -> (data out=w934:string, error out=w929:errorcluster, 3:w930:refnum<k16>)  [unwired: 2 out]
    n389 = Wait Until Next ms Multiple(millisecond multiple=u32 500) -> ()  [unwired: 1 out]
    n390 = case shown="No Error" w929 {
      tunnel: w929 -> [w938 w952]
      tunnel: w934 -> [w942 _]
      tunnel: [w937 w952] -> w931
      frame No Error {
        n391 = call <vilib>:"Find Item.vi"("$Path or Item Name"="Facade", "JSON"=w942) -> ("<JSON>"=w939:string, "Found"=w940:bool)  [unwired: 6 in, 2 out]
        n392 = case shown="True" w940 {
          tunnel: w939 -> [_ w951]
          tunnel: w938 -> [w945 w950]
          tunnel: [w945 w949] -> w937
          tunnel: [w944 w946] -> w941
          frame False {
            n393 = local read "P_pv_facade"() -> (w944:dbl)
          }
          frame True {
            n394 = Unflatten From JSON(JSON string=w951, type and defaults=T32 {"Info"={"Resource"="Zenone", "Problem"=FALSE, "Timestamp"=0.0}, "Data"={"P"=0.0, "Q"=0.0, "Pset"=0.0, "Qset"=0.0}} ("Cluster"), error in (no error)=w950) -> (value=w947:T32, error out=w949:errorcluster)  [unwired: 4 in]
            n395 = Unbundle By Name(w947) -> ("Data.P"=w946:dbl)
          }
        }
        n396 = local write "P_pv_facade"(w941) -> ()
      }
      frame Error {
      }
    }
  }
  n397 = while {
    tunnel: w73 -> [w962]
    tunnel: w72 -> [w961]
    tunnel: [w960] -> w75
    tunnel: [w959] -> w74
    stop <- w956 stop-if-true
    (unwired) i64 0 ("Iteration Duration")
    n398 = Wait Until Next ms Multiple(millisecond multiple=u32 100) -> ()  [unwired: 1 out]
    n399 = UDP Read(connection ID=w962, max size (548)=2000, timeout ms (25000)=50, 8:w961) -> (data out=w963:string, error out=w958:errorcluster, 3:w959:refnum<k16>)  [unwired: 2 out]
    n400 = call <vilib>:"Is Empty.vi"("JSON"=w963) -> ("Empty"=w964:bool)  [unwired: 4 in]
    n401 = Not(x=w964) -> (.not. x?=→"iOPF data":bool)
    n402 = case shown="Error .." w958 {
      tunnel: w958 -> [w969 w972]
      tunnel: w963 -> [w968 _]
      tunnel: [w970 w972] -> w960
      tunnel: [w966 w971] -> w955
      frame No Error {
        n403 = Unflatten From JSON(JSON string=w968, type and defaults=T17 {"Info"={"Resource"="Zenone", "Problem"=0.0, "Timestamp"=0.0}, "Data"={"Operation_mode"="Grid connected", "solution_feasible"=0.0, "Optimal_slack"="AFE 1", "setpoints"=[], "upper_layer_grid_info"={"Frequency"=0.0, "Angle"=0.0, "Magnitude"=0.0}, "SC_soc"=0.0, "PV"={"perun"=0.0, "solarmax"=0.0, "facade"=0.0, "emul4"=0.0, "emul5"=0.0, "emul6"=0.0, "emul7"=0.0}, "P_pv_facade"=0.0}} ("IN iOPF"), error in (no error)=w969) -> (value=w966:T17, error out=w970:errorcluster)  [unwired: 4 in]
      }
      frame Error {
        n404 = local read "IN iOPF"() -> (w971:T17)
      }
    }
    n405 = local read "Stop"() -> (w956:bool)
    n406 = local write "IN iOPF"(w955) -> ()
  }
  n407 = while {
    tunnel: w56 -> [w975]
    tunnel: w55 -> [w974]
    tunnel: w51 -> [w979]
    tunnel: w50 -> [w976]
    tunnel: [w978] -> w53
    tunnel: [w977] -> w52
    stop <- w986 stop-if-true
    n408 = local read "Zenone_Q"() -> (w982:dbl)
    n409 = local read "Zenone_P"() -> (w983:dbl)
    n410 = local read "setpoints"() -> (w985:dbl[])
    n411 = Wait Until Next ms Multiple(millisecond multiple=u32 500) -> ()  [unwired: 1 out]
    n412 = call "Setpoint.vi"("ZENONE.Q_set [kVAr]"=w982, "ZENONE.P_set [kW]"=w983, "setpoints IN"=w985) -> ("OUT"=w980:T35)  [unwired: 8 in]
    n413 = Flatten To JSON(anything=w980) -> (JSON string=w984:string)  [unwired: 2 in, 1 out]
    n414 = case shown="True" "Send sp AC?" {
      tunnel: w984 -> [_ w996]
      tunnel: w979 -> [w988 w993]
      tunnel: [w988 w995] -> w978
      tunnel: [w987 w994] -> w977
      tunnel: w976 -> [w987 w992]
      tunnel: w975 -> [_ w990]
      tunnel: w974 -> [_ w989]
      frame False {
      }
      frame True {
        n415 = UDP Write(address=w989, port or service name=w990, connection ID=w993, data in=w996, 8:w992, 9:50 ("timeout ms (25000)")) -> (error out=w994:errorcluster, 3:w995:refnum<k16>)
      }
    }
    n416 = local read "Stop"() -> (w986:bool)
  }
  n417 = while {
    tunnel: w63 -> [w1008]
    tunnel: w71 -> [w1007]
    tunnel: w68 -> [w1005]
    tunnel: w67 -> [w1004]
    tunnel: [w1003] -> w70
    tunnel: [w1002] -> w69
    stop <- w1001 stop-if-true
    n418 = local read "OUT iOPF"() -> (w998:T17)
    n419 = Flatten To JSON(anything=w998, error in (no error)=w1004) -> (JSON string=w1006:string, 11:w1000:errorcluster)  [unwired: 1 in]
    n420 = UDP Write(address=w1007, port or service name=w1008, connection ID=w1005, data in=w1006, 8:w1000, 9:50 ("timeout ms (25000)")) -> (error out=w1002:errorcluster, 3:w1003:refnum<k16>)
    n421 = local read "Stop"() -> (w1001:bool)
    n422 = Wait Until Next ms Multiple(millisecond multiple=u32 100) -> ()  [unwired: 1 out]
  }
  n423 = UDP Close(connection ID=w17, 8:w18) -> ()  [unwired: 2 out]
  n424 = UDP Close(connection ID=w39, 8:w38) -> ()  [unwired: 2 out]
  n425 = UDP Close(connection ID=w70, 8:w69) -> ()  [unwired: 2 out]
  n426 = UDP Close(connection ID=w43, 8:w44) -> ()  [unwired: 2 out]
  n427 = UDP Close(connection ID=w74, 8:w75) -> ()  [unwired: 2 out]
  n428 = UDP Close(connection ID=w53, 8:w52) -> ()  [unwired: 2 out]
  n429 = UDP Close(connection ID=w61, 8:w62) -> ()  [unwired: 2 out]
  n430 = node-c288(w4) -> ()  [unwired: 1 out]
